vi "GUI_Cameras.vi"() -> ()   [LabVIEW 2020]
uses:
  Shared/GUI_Template/GUI_master/tcp_new_data_event.ctl
  Shared/GUI_Template/GUI_master/tcp new data cluster.ctl
  color tables/image color table presets.ctl
  Controls/Crosshair type def.ctl
  Controls/IMAQ control.ctl
  <vilib>/vision/Image Controls.llb/IMAQ Image.ctl
  Controls/Image Processing Controls.ctl
  Controls/GUI_running average centroid overlay.ctl
  Controls/Image Analysis Controls.ctl
  <vilib>/Utility/miscctls.llb/LVRectTypeDef.ctl
  <userlib>/_OpenG.lib/comparison/comparison.llb/Boolean Changed__ogtk.vi
  <vilib>/vision/NI_Vision_Development_Module.lvlib
panel:
  in  "stop":bool
  in  "Maximize!!":bool
  out "image::1":T1(plugin-control) caption="HPD_CCD"
  out "tcp data event":T2
  in  "Tab Control":T3(tab)
  out "Timestamp":timestamp format="%<%I:%M:%S%3u %p>T"
  in  "Max count":T4(ring)
  in  "Size & Tolerance":T5={"X Size"=5, "Y Size"=5, "% Tolerance"=100} {"Y Size" min=1 max=8; "X Size" min=1 max=8}
  in  "Clear ROI":bool caption="draw Xhair"
  in  "Set ROI":bool caption="draw Xhair"
  in  "LowPass":bool
  out "Max Counts":dbl(slide) scale=0.0..255.0
  in  "Color table":T6=enum."Rainbow"
  out "Rate (Hz)":sgl
  in  "analysis::1":bool caption="Analysis"
  in  "Scale":bool
  in  "Autoscale":bool
  in  "trigger::1":bool caption="Trigger"
  in  "save::1":bool caption="Save"
  in  "Scale":bool caption="Beep if Sat"
  in  "PerspectiveCorrectGUI::1":bool caption="Perspective"
  in  "roi.offsetY::1":u32 caption="ROI:OffsetY" max=1000
  in  "roi.offsetX::1":u32 caption="ROI:OffsetX" max=1000
  in  "roi.height::1":u32 caption="ROI:Height" min=1 max=3000
  in  "roi.width::1":u32 caption="ROI.Width" min=1 max=3000
  in  "SpatialCalibration::1":dbl caption="um/pix" min=0.0 max=9999999.0
  in  "Sat Level":sgl=255.0
  in  "triggerdelay::1":dbl caption="Triggerdelay" min=0.0 max=0.09
  in  "exposure::1":dbl=0.52 caption="Exposure" min=3.8e-05 max=1.0
  in  "gain::1":dbl caption="Gain" min=0.0 max=240.0
  in  "scale factor":dbl=2.0 caption="Scale factor"
  out "UDP error message":string caption="Device Errors"
  out "Perspective error":bool
  out "LastUpdate(s)":dbl format="%#_3g"
  in  "Type of Symmetry":T7(ring)
  in  "Rotate 2":bool caption="Flip"
  in  "Angle":dbl
  in  "Rotate":bool
  in  "BG Bit depth":string="12"
  in  "Subtract background":bool
  in  "BackgroundPath::1":path caption="BackgroundPath"
  in  "PerspectivePath::1":path caption="Perspective Calibration File Path"
  in  "AnalysisROITop::1":u32 caption="Top" max=2500
  in  "AnalysisROILeft::1":u32 caption="Left" max=2500
  in  "AnalysisROIBottom::1":u32 caption="Bottom" max=3000
  in  "AnalysisROIRight::1":u32 caption="Right" max=2500
  in  "Set Analysis ROI":bool caption="draw Xhair"
  in  "AnalysisROI::1":bool caption="AnalysisROI"
  in  "Draw From Centroid 2":bool=TRUE caption="draw Xhair"
  in  "Draw From\n Centroid 1":bool=TRUE caption="draw Xhair"
  in  "Crosshair.Label2::1":string="HPD_CCD" caption="CrosshairLabel2"
  in  "Crosshair.Label1::1":string="HPD_CCD" caption="CrosshairLabel1"
  in  "Target2.X::1":dbl caption="Target2X" min=0.0 max=2000.0
  in  "Target2.Y::1":dbl caption="Target2Y" min=0.0 max=2000.0
  in  "draw Xhair 2":bool caption="draw Xhair"
  in  "Target2Size.X::1":dbl=20.0 caption="Size2 x" min=0.0 max=2000.0
  in  "Target2Size.Y::1":dbl=20.0 caption="Size2 y" min=0.0 max=2000.0
  in  "Crosshair 2\nColor":u32(colorbox)=1250067
  in  "Crosshair 2Thickness":i32=1 caption="Crosshair 2\nThickness" min=0 max=2000
  in  "Overlay\nCentroid":T8={"draw Xhair 2"=FALSE, "Size x"=20.0, "Size y"=20.0, "# images to average"=20, "Centroid \nOverlay Color"=13435100} {"# images to average" min=0 max=2000; "Size y" min=0.0 max=2000.0; "Size x" min=0.0 max=2000.0}
  in  "Target.X::1":dbl caption="TargetX" min=0.0 max=2000.0
  in  "Target.Y::1":dbl caption="TargetY" min=0.0 max=2000.0
  in  "draw Xhair":bool=TRUE
  in  "TargetSize.X::1":dbl=20.0 caption="Size x" min=2.0 max=3000.0
  in  "TargetSize.Y::1":dbl=20.0 caption="Size y" min=2.0 max=3000.0
  in  "Crosshair\nColor":u32(colorbox)=1250067
  in  "Crosshair Thickness":i32=1 caption="Crosshair\nThickness" min=0 max=2000
  in  "GUI Crosshair":T9={"Draw"=FALSE, "Target"={"x"=0.0, "y"=0.0}, "Size"={"x"=20.0, "y"=20.0}, "Angle"=0.0, "Color"=1250067, "Thickness"=1, "CrosshairLabel"=""} {"Thickness" max=0; "Angle" format="%#_13g"; "Size"."y" min=0.0 max=0.0; "Size"."x" min=0.0 max=0.0}
  out "2ndmomW0y45::1":dbl caption="2ndmomW0y45" min=0.0 max=999999.0
  out "2ndmomW0x45::1":dbl caption="2ndmomW0x45" min=0.0 max=999999.0
  out "2ndmomW0y::1":dbl caption="2ndmomW0y" min=0.0 max=999999.0
  in  "Tab Control 2":enum32{"Mean", "Histogram", "Lineout"}(tab)
  out "Chart":dbl[][](graph)
  out "histogram":T10(graph)
  out "Mean Value":sgl format="%.2f"
  out "lineout":cluster{"x0":sgl, "dx":sgl, "Pixels Line":sgl[]}(graph)
  in  "GUI_Analysis":bool
  out "FWHMx (um)":dbl
  out "FWHMy (um)":dbl
  out "2ndmomW0x::1":dbl caption="2ndmomW0x" min=0.0 max=999999.0
  in  "FWHMx::1":dbl caption="FWHMx" min=0.0 max=999999.0
  in  "FWHMy::1":dbl caption="FWHMy" min=0.0 max=999999.0
  in  "centroidx::1":dbl caption="Centroidx" min=0.0 max=0.0
  in  "centroidy::1":dbl caption="Centroidy" min=0.0 max=0.0
  out "meancounts::1":dbl caption="MeanCounts" min=0.0 max=999999999.0
  in  "maxcounts::1":dbl caption="MaxCounts" min=0.0 max=999999999.0
  in  "acq_timestamp::1":dbl caption="acq_timestamp" min=0.0 max=0.0
  in  "localsavingpath::1":path caption="LocalSavingPath"
  in  "GUIdevice 1":string="HPD_CCD"
  in  "Hide controls":bool
  out "Current State":string
  out "ms since last display":u32
  out "process time":u32
  out "Custom Data Out":string
  out "Image Different?":bool
  in  "MeanCountsRaw::1":dbl caption="MeanCountsRaw" min=0.0 max=0.0
  out "Image (IMAQ)":T1(plugin-control)
  # "Set Crosshair\nto Centroid"
  # "Mean"
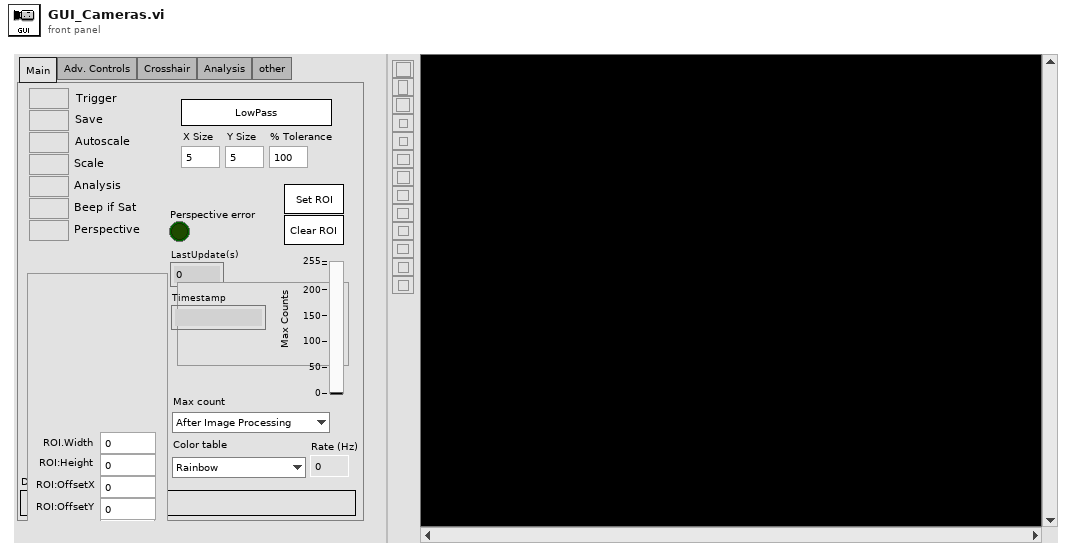
[diagram p1: front panel]
types:
  T1 = typedef "IMAQ Image.ctl" = refnum<image>
  T2 = typedef "tcp_new_data_event.ctl" = refnum<user-event>
  T3 = enum32{"Main", "Adv. Controls", "Crosshair", "Analysis", "other"}
  T4 = enum16{"After Image Processing", "Before Image Processing"}
  T5 = cluster{"X Size":i32, "Y Size":i32, "% Tolerance":i32}
  T6 = typedef "image color table presets.ctl" = enum16{"Greyscale", "Binary", "Gradient", "Rainbow", "Temperature", "enhance low", "blue yellow red", "BYR enhance low", "white blue yellow", "BWR enhance low", "make a new one"}
  T7 = enum16{"Horizontal", "Vertical", "Central", "1st Diagonal", "2nd Diagonal"}
  T8 = cluster{"draw Xhair 2":bool, "Size x":dbl, "Size y":dbl, "# images to average":i32, "Centroid \nOverlay Color":u32}
  T9 = typedef "Crosshair type def.ctl" = cluster{"Draw":bool, "Target":cluster{"x":dbl, "y":dbl}, "Size":cluster{"x":dbl, "y":dbl}, "Angle":dbl, "Color":u32, "Thickness":u8, "CrosshairLabel":string}
  T10 = cluster{"Starting Value":sgl, "Incremental Value":sgl, "Histogram":u32[]}
  T11 = enum32{"Invalid", "Standard", "Closed", "Hidden", "Minimized", "Maximized"}
  T12 = enum32{"invalid app kind", "Development System", "Run Time System", "Student Edition", "Embedded LabVIEW", "Evaluation", "Custom"}
  T13 = typedef "tcp new data cluster.ctl" = cluster{"EventEnum":enum16{"new data", "connection status update"}, "Device name":string}
  T14 = typedef "GUI_running average centroid overlay.ctl" = cluster{"CentroidX array":dbl[], "CentroidY array":dbl[], "CentroidX":dbl, "CentroidY":dbl, "# images to average":i32, "Crosshair":T9}
  T15 = cluster{"2ndmomW0y45::1":dbl, "2ndmomW0x45::1":dbl, "2ndmomW0y::1":dbl, "2ndmomW0x::1":dbl}
  T16 = cluster{"SpatialCalibration":dbl, "FWHMx":dbl, "FWHMy":dbl, "Analysis":bool}
  T17 = cluster{"LowPass":bool, "Size & Tolerance":cluster{"X Size":i32, "Y Size":i32, "% Tolerance":i32}}
  T18 = cluster{"Global Rectangle":i32[], "Contours":cluster{"Contour Type":u32, "ROI Type":u32, "Points":i32[]}[]}
  T19 = typedef "IMAQ Rectangle" = cluster{"Left":i32, "Top":i32, "Right":i32, "Bottom":i32, "Rotation":dbl}
  T20 = typedef "IMAQ control.ctl" = cluster{"Image SM":T1, "valid image":bool, "X resolution":i32, "Y resolution":i32, "Image Area":cluster{"Width":u32, "Height":u32}, "zoom to fit":bool, "Image Center":cluster{"X":u32, "Y":u32}, "Max count":dbl}
  T21 = typedef "Image Processing Controls.ctl" = cluster{"Crosshair IN":T9, "Autoscale":bool, "Scale":cluster{"scale factor":dbl, "Scale":bool}, "Lowpass IN":cluster{"LowPass":bool, "Size & Tolerance":cluster{"X Size":i32, "Y Size":i32, "% Tolerance":i32}}, "Image":T1, "GUI_centroid overlay":T14, "GUI Crosshair":T9, "Crosshair2 IN":T9, "calibration image":T1, "Perspective correection":bool, "Background image":T1, "Subtract background":bool, "Rotate Image":cluster{"Rotate":bool, "Rotation Angle":dbl}, "Flip Image":cluster{"Ring":u16, "Flip":bool}}
  T22 = typedef "Image Analysis Controls.ctl" = cluster{"Analysis":cluster{"IN":cluster{"SpatialCalibration":dbl, "FWHMx":dbl, "FWHMy":dbl, "Analysis":bool}, "OUT":cluster{"FWHMx (um)":dbl, "FWHMy (um)":dbl}}, "Histogram OUT":cluster{"histogram":cluster{"Starting Value":sgl, "Incremental Value":sgl, "Histogram":u32[]}, "Mean Value Graph":sgl, "Mean Value":sgl}, "Lineout":cluster{"IN":cluster{"ROI":cluster{"Global Rectangle":i32[], "Contours":cluster{"Contour Type":u32, "ROI Type":u32, "Points":i32[]}[]}}, "OUT":cluster{"lineout":cluster{"x0":sgl, "dx":sgl, "Pixels Line":sgl[]}, "Centroid":cluster{"X Centroid":sgl, "Y Centroid":sgl}, "Max Counts":cluster{"Max":sgl, "Color":u32}}}, "Image":T1, "variables":cluster{"2ndmomW0y45::1":dbl, "2ndmomW0x45::1":dbl, "2ndmomW0y::1":dbl, "2ndmomW0x::1":dbl}}
  T23 = typedef "LVRectTypeDef.ctl" = cluster{"Left":i16, "Top":i16, "Right":i16, "Bottom":i16}
  T24 = cluster{"Core":cluster{"Current VI Reference":refnum<vi>, "Close Panel on Exit?":bool}, "tcp connections":refnum<k5>[], "subscribe messages":string[], "Image Data":T20, "Image Process":T21, "Image Analysis":T22, "FP":cluster{"size":T23, "Resize Image":bool}, "Max count":dbl, "Max count before Image Processing":dbl, "Supergui":cluster{"image::1":T1, "STOP queue":refnum<queue>, "SuperGUI ref":refnum<vi>}, "Graph":dbl[][], "New Image":T1, "All Devices":string[], "PerspectivePath":path, "Old Timestamp":dbl}
  T25 = typedef "Image Type" = u32
  T26 = cluster{"image::1":T1, "STOP queue":refnum<queue>, "SuperGUI ref":refnum<vi>}
  T27 = cluster{"Current VI Reference":refnum<vi>, "Close Panel on Exit?":bool}
  T28 = cluster{"histogram":u32[], "Minimal Value":sgl, "Maximal Value":sgl, "Starting Value":sgl, "Interval Width":sgl, "Mean Value":sgl, "Standard  Variation":sgl, "Area (pixels)":i32}
  T29 = cluster{"TargetSize.X::1":dbl, "TargetSize.Y::1":dbl}
  T30 = cluster{"Target2Size.X::1":dbl, "Target2Size.Y::1":dbl}
  T31 = cluster{"Type of Symmetry":enum16{"Horizontal", "Vertical", "Central", "1st Diagonal", "2nd Diagonal"}, "Rotate 2":bool}
  T32 = cluster{"lineout":cluster{"x0":sgl, "dx":sgl, "Pixels Line":sgl[]}, "Centroid":cluster{"X Centroid":sgl, "Y Centroid":sgl}, "Max Counts":cluster{"Max":sgl, "Color":u32}}
  T33 = cluster{"histogram":cluster{"Starting Value":sgl, "Incremental Value":sgl, "Histogram":u32[]}, "Mean Value Graph":sgl, "Mean Value":sgl}
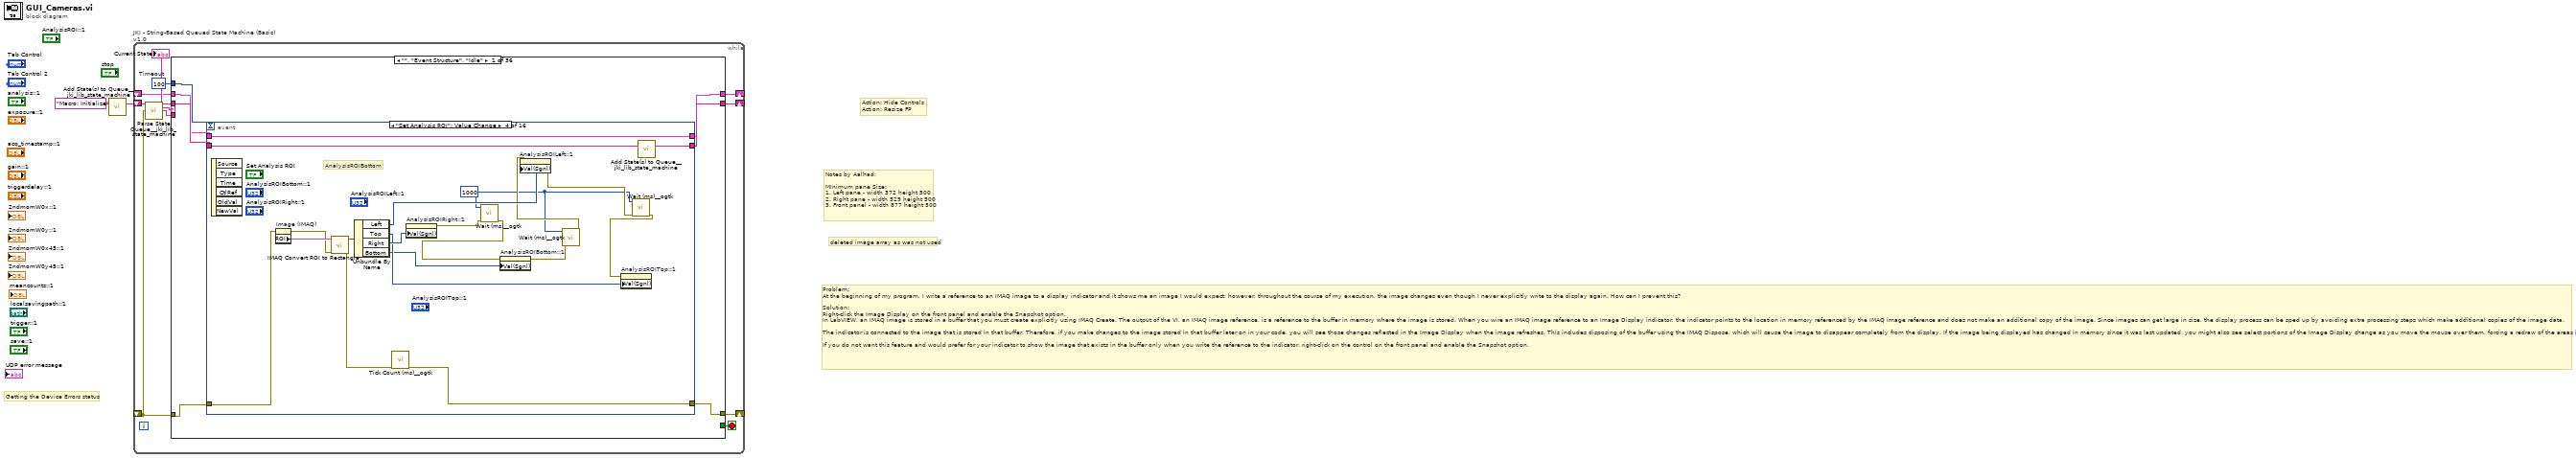
[diagram p0: block diagram]
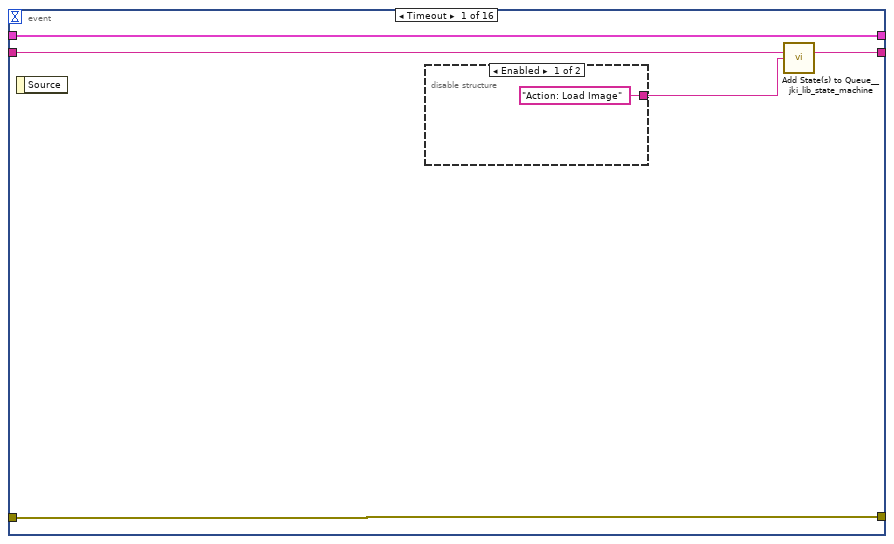
[diagram p2: hidden frame]
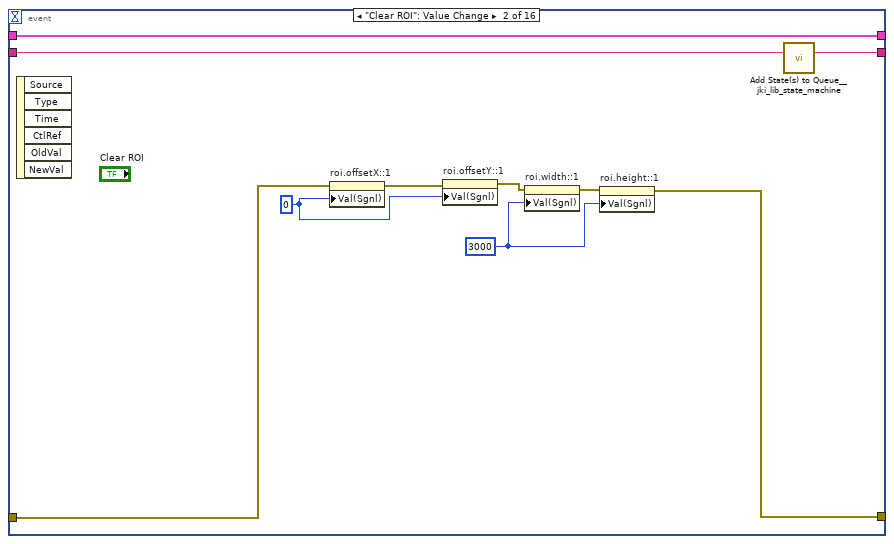
[diagram p4: hidden frame]
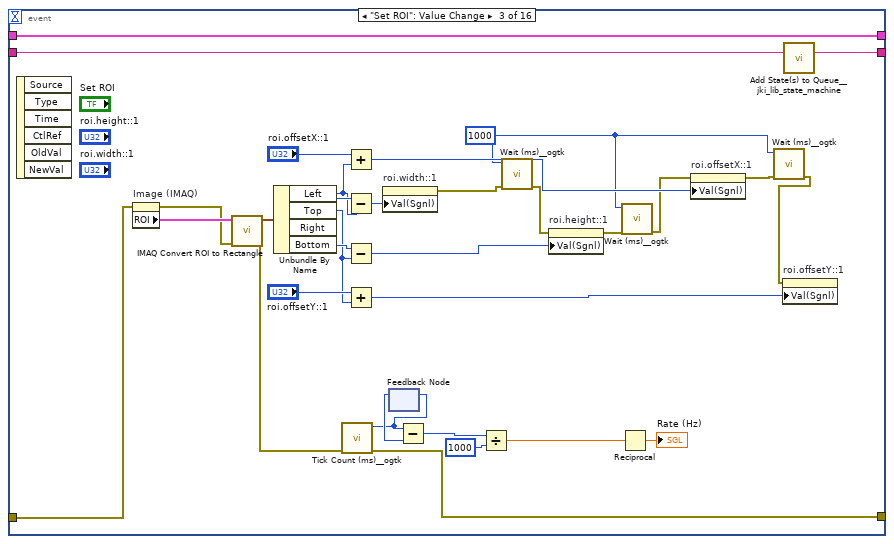
[diagram p5: hidden frame]
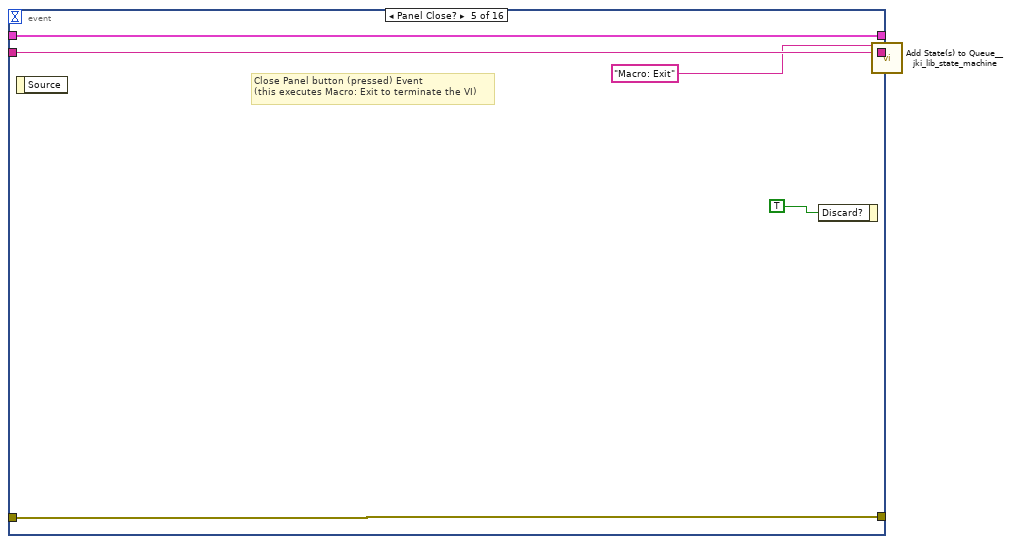
[diagram p6: hidden frame]
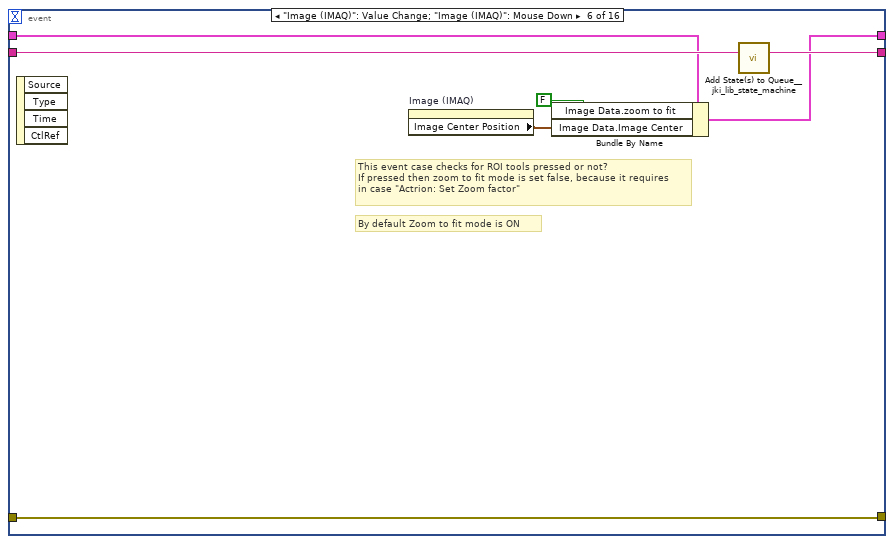
[diagram p7: hidden frame]
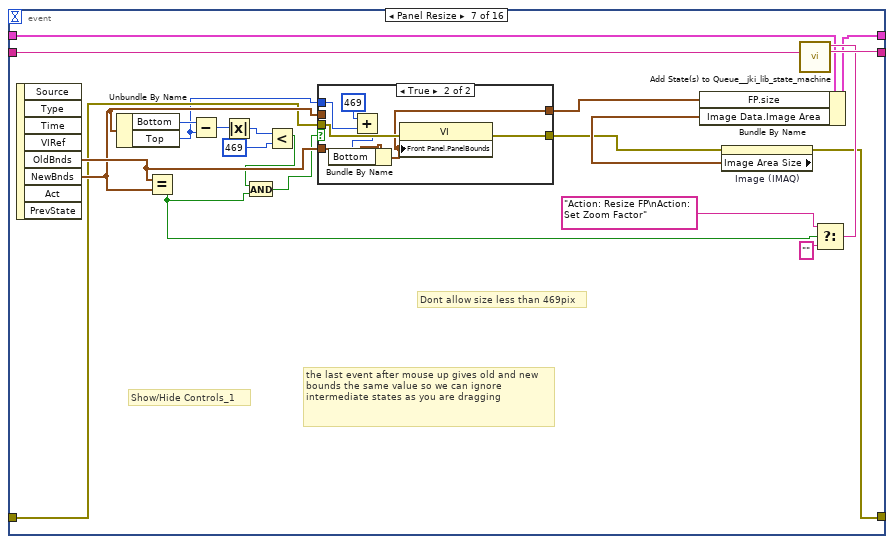
[diagram p8: hidden frame]
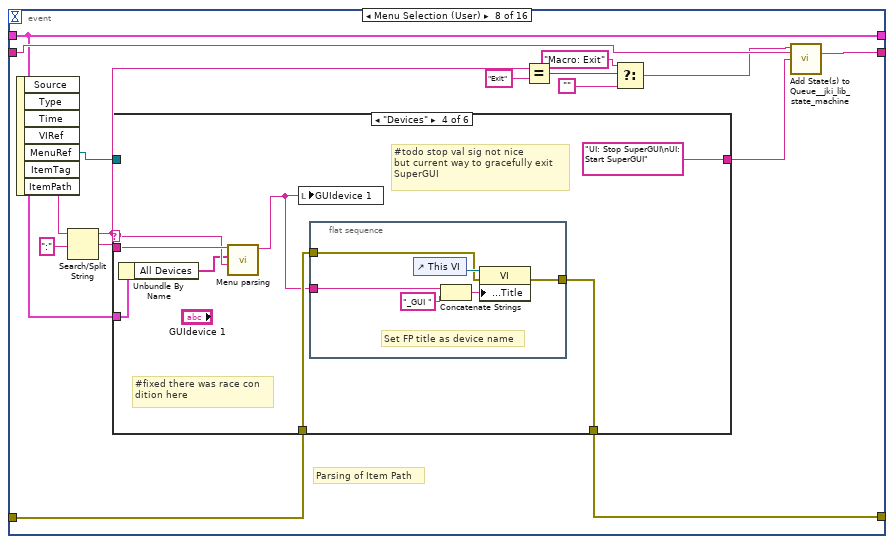
[diagram p10: hidden frame]
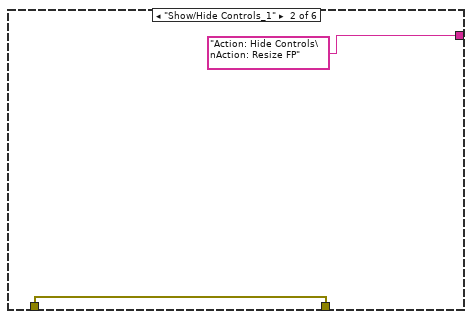
[diagram p12: hidden frame]
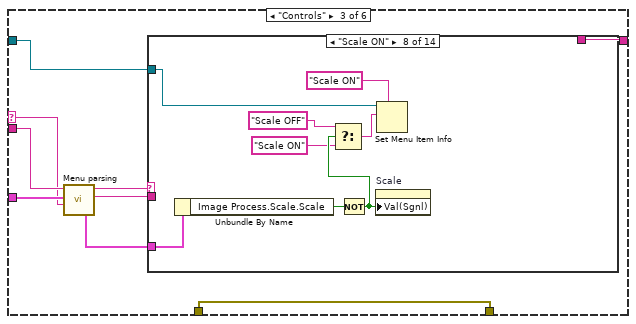
[diagram p13: hidden frame]
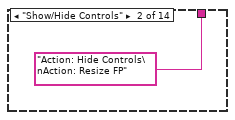
[diagram p15: hidden frame]
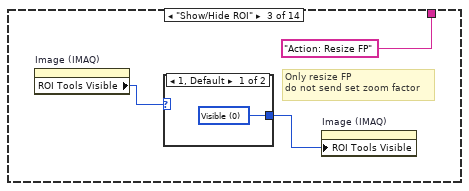
[diagram p16: hidden frame]
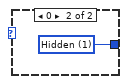
[diagram p17: hidden frame]
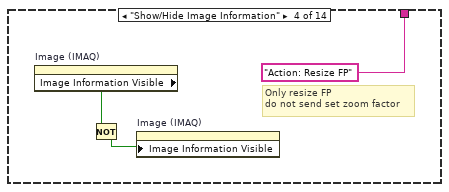
[diagram p18: hidden frame]
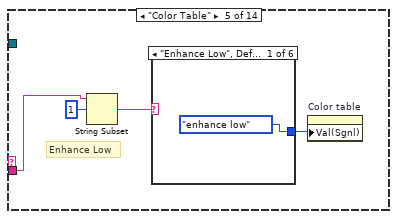
[diagram p19: hidden frame]
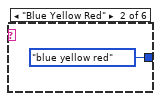
[diagram p20: hidden frame]
diagram:
  # "Getting the Device Errors status"
  # "Notes by Aalhad:\n\nMInimum pane Size:\n1. Left pane - width 372 height 500\n2. Right pane - width 529 height 500\n3. Front panel - width 877 height 500"
  # "deleted image array as was not used"
  # "Problem: \nAt the beginning of my program, I write a reference to an IMAQ image to a display indicator and it shows me an image I would expect; however, throughout the course of my execution, the image changes even though I never explicitly write to the display again. How can I prevent this?\n\nSolution: \nRight-click the Image Display on the front panel and enable the Snapshot option.\nIn LabVIEW, an IMAQ image is stored in a buffer that you must create explicitly using IMAQ Create. The output of the VI, an IMAQ image reference, is a reference to the buffer in memory where the image is stored. When you wire an IMAQ image reference to an Image Display indicator, the indicator points to the location in memory referenced by the IMAQ image reference and does not make an additional copy of the image. Since images can get large in size, the display process can be sped up by avoiding extra processing steps which make additional copies of the image data.\n\nThe indicator is connected to the image that is stored in that buffer. Therefore, if you make changes to the image stored in that buffer later on in your code, you will see those changes reflected in the Image Display when the image refreshes. This includes disposing of the buffer using the IMAQ Dispose, which will cause the image to disappear completely from the display. If the image being displayed has changed in memory since it was last updated, you might also see select portions of the Image Display change as you move the mouse over them, forcing a redraw of the areas it passes through.\n\nIf you do not want this feature and would prefer for your indicator to show the image that exists in the buffer only when you write the reference to the indicator, right-click on the control on the front panel and enable the Snapshot option."
  # "Action: Hide Controls\nAction: Resize FP"
  n1 = call <vilib>:"Add State(s) to Queue__jki_lib_state_machine.vi"("State(s) in (\"\")"="Macro: Initialize") -> ("States Out"=w2:string)  [unwired: 14 in]
  n2 = while "JKI - String-Based Queued State Machine (Basic) v1.0" {
    shift-right: [w6] -> _
    shift-left: _ -> [w5]
    shift-right: [w9] -> _
    shift-left: _ -> [w3]
    shift-right: [w8] -> _
    shift-left: w2 -> [w10]
    stop <- w7 stop-if-true
    w4 = 100  # Timeout
    n3 = call <vilib>:"Parse State Queue__jki_lib_state_machine.vi"("State Queue"=w10, "Error In (no error)"=w3) -> ("Remaining States"=w12:string, "Current State"=w13:string, "Arguments"=w11:string)  [unwired: 11 in]
    "Current State" <- w13
    n4 = case shown="\"\", \"Event Structure\", \"Idle\"" w13 {
      selector: w13 -> [_ _ w352 _ _ _ _ _ _ _ _ _ _ _ _ _ _ _ _ _ _ _ _ _ _ _ _ _ _ _ _ _ _ _ _ _]
      tunnel: w12 -> [w20 w351 w356 w374 w382 w397 w401 w428 w437 w444 w461 w473 w478 w514 w539 w570 w592 w602 w637 w642 w647 w659 w663 w671 w703 w740 w764 w805 w831 w901 w923 w952 w989 w1005 w1023 w1048]
      tunnel: w11 -> [_ _ _ _ _ _ _ _ _ _ _ _ _ _ _ _ w587 w597 _ _ _ _ _ _ _ _ _ _ _ _ _ _ _ _ _ _]
      tunnel: w5 -> [w18 w348 w354 w366 w380 w395 w398 _ w434 w441 w455 w468 w479 w515 w538 w553 w590 w598 w634 w639 w644 w657 w660 w664 w697 w725 w771 w804 w835 w862 w921 w944 w972 w1006 w1020 w1037]
      tunnel: [w17 w349 w358 w371 w375 w394 w399 w425 w431 w442 w459 w462 w476 w511 w534 w557 w588 w599 w635 w640 w645 w651 w661 w665 w699 w727 w765 w807 w836 w900 w922 w930 w966 w1002 w1017 w1029] -> w9
      tunnel: w3 -> [w16 w349 w357 w371 w376 w394 w399 w425 w430 w442 w459 w469 w477 w512 w533 w554 w589 w600 w635 w640 w645 w651 w661 w669 w701 w734 w766 w824 w833 w900 w922 w948 w965 w1003 w1018 w1027]
      tunnel: [w19 w350 w355 w373 w381 w396 w400 w427 w436 w443 w460 w473 w478 w514 w539 w570 w591 w601 w636 w641 w646 w658 w662 w670 w702 w739 w763 w806 w831 w901 w923 w952 w989 w1005 w1023 w1047] -> w8
      tunnel: [_ _ _ _ _ TRUE _ _ _ _ _ _ _ _ _ _ _ _ _ _ _ _ _ _ _ _ _ _ _ _ _ _ _ _ _ _] -> w7
      tunnel: [w15 w348 w354 w372 w380 w395 w398 w426 w434 w441 w454 w467 w479 w515 w538 w556 w590 w598 w634 w639 w644 w657 w660 w668 w700 w726 w770 w803 w834 w899 w920 w949 w972 w1006 w1020 w1037] -> w6
      tunnel: w4 -> [w14 _ _ _ _ _ _ _ _ _ _ _ _ _ _ _ _ _ _ _ _ _ _ _ _ _ _ _ _ _ _ _ _ _ _ _]
      frame "", "Event Structure", "Idle" {
        n5 = event shown="[3] \"Set Analysis ROI\": Value Change" {
          selector: _ -> [_ _ _ _ _ _ _ _ _ _ _ _ _ _ _ _]
          dyn-events: _ -> [_ _ _ _ _ _ _ _ _ _ _ _ _ _ _ _]
          timeout: w14 -> [_ _ _ _ _ _ _ _ _ _ _ _ _ _ _ _]
          tunnel: w20 -> [w25 w36 w68 w88 w94 w100 w122 w140 w280 w298 w304 w309 w315 w331 w339 w347]
          tunnel: [w24 w35 w67 w87 w93 w101 w123 w138 w279 w297 w303 w309 w315 w331 w339 w347] -> w19
          tunnel: w18 -> [w21 w34 w66 w86 w91 w99 w118 w133 w286 w300 w306 w310 w316 w326 w337 w345]
          tunnel: [w23 w27 w44 w77 w92 w98 w106 w135 w281 w299 w305 w308 w311 w330 w338 w346] -> w17
          tunnel: w16 -> [w23 w28 w45 w78 w92 w98 w107 w136 w282 w299 w305 w308 w312 w330 w338 w346]
          tunnel: [w21 w34 w66 w86 w91 w97 w117 w133 w286 w300 w306 w310 w316 w325 w337 w345] -> w15
          event Timeout {
            n6 = event-data() -> ()  [unwired: 1 in, 1 out]
            n7 = disable-structure shown="Enabled" {
              disable-tunnel: ["Action: Load Image" ("State(s) in Front (\"\")") _] -> w22
              frame Enabled {
              }
              frame Disabled {
              }
            }
            n8 = call <vilib>:"Add State(s) to Queue__jki_lib_state_machine.vi"("State(s) in (\"\")"=w25, "State(s) at Back (\"\")"=w22) -> ("States Out"=w24:string)  [unwired: 13 in]
          }
          event "Clear ROI": Value Change {
            w31 = 3000
            w33 = 0
            n9 = event-data() -> ()  [unwired: 1 in, 6 out]
            n10 = property on="roi.offsetX::1" class="DigNum (strict)"(error in=w28, "Val(Sgnl)"=w33) -> (error out=w32:errorcluster)  [unwired: 1 in, 1 out]
            n11 = property on="roi.offsetY::1" class="DigNum (strict)"(error in=w32, "Val(Sgnl)"=w33) -> (error out=w30:errorcluster)  [unwired: 1 in, 1 out]
            n12 = property on="roi.width::1" class="DigNum (strict)"(error in=w30, "Val(Sgnl)"=w31) -> (error out=w29:errorcluster)  [unwired: 1 in, 1 out]
            n13 = property on="roi.height::1" class="DigNum (strict)"(error in=w29, "Val(Sgnl)"=w31) -> (error out=w27:errorcluster)  [unwired: 1 in, 1 out]
            n14 = call <vilib>:"Add State(s) to Queue__jki_lib_state_machine.vi"("State(s) in (\"\")"=w36) -> ("States Out"=w35:string)  [unwired: 14 in]
          }
          event "Set ROI": Value Change {
            w38 = u32 1000 ("milliseconds to wait")
            n15 = event-data() -> ()  [unwired: 1 in, 6 out]
            n16 = property on="Image (IMAQ)" class="ImageControl"(error in=w45) -> (error out=w47:errorcluster, "ROI"=w64:T18)  [unwired: 1 in, 1 out]
            n17 = call "IMAQ Convert ROI to Rectangle"("error in (no error)"=w47, "ROI Descriptor"=w64) -> ("error out"=w46:errorcluster, "Rectangle"=w65:T19)  [unwired: 7 in]
            n18 = Unbundle By Name(w65) -> ("Left"=w58:i32, "Top"=w55:i32, "Right"=w59:i32, "Bottom"=w56:i32)
            n19 = call <userlib>:"Tick Count (ms)__ogtk.vi"("error in (no error)"=w46) -> ("error out"=w44:errorcluster, "millisecond timer value"=w52:u32)  [unwired: 9 in]
            n20 = Add(x="roi.offsetX::1", y=w58) -> (x+y=w62:u32)
            n21 = Subtract(x=w59, y=w58) -> (x-y=w57:i32)
            n22 = Subtract(x=w56, y=w55) -> (x-y=w54:i32)
            n23 = Add(x="roi.offsetY::1", y=w55) -> (x+y=w60:u32)
            n24 = property on="roi.width::1" class="DigNum (strict)"("Val(Sgnl)"=w57) -> (error out=w43:errorcluster)  [unwired: 2 in, 1 out]
            n25 = feedback #1() -> (w53:u32)  [unwired: 1 in]
            n26 = feedback-in #1(w52) -> ()
            n27 = Subtract(x=w52, y=w53) -> (x-y=w51:u32)
            n28 = Divide(x=w51, y=u32 1000) -> (x/y=w49:dbl)
            n29 = call <userlib>:"Wait (ms)__ogtk.vi"("error in (no error)"=w43, "milliseconds to wait"=w38) -> ("error out"=w42:errorcluster)  [unwired: 8 in, 1 out]
            n30 = property on="roi.height::1" class="DigNum (strict)"(error in=w42, "Val(Sgnl)"=w54) -> (error out=w41:errorcluster)  [unwired: 1 in, 1 out]
            n31 = Reciprocal(x=w49) -> (1/x=→"Rate (Hz)":dbl)
            n32 = call <userlib>:"Wait (ms)__ogtk.vi"("error in (no error)"=w41, "milliseconds to wait"=w38) -> ("error out"=w40:errorcluster)  [unwired: 8 in, 1 out]
            n33 = property on="roi.offsetX::1" class="DigNum (strict)"(error in=w40, "Val(Sgnl)"=w62) -> (error out=w39:errorcluster)  [unwired: 1 in, 1 out]
            n34 = call <userlib>:"Wait (ms)__ogtk.vi"("error in (no error)"=w39, "milliseconds to wait"=w38) -> ("error out"=w37:errorcluster)  [unwired: 8 in, 1 out]
            n35 = property on="roi.offsetY::1" class="DigNum (strict)"(error in=w37, "Val(Sgnl)"=w60) -> ()  [unwired: 1 in, 2 out]
            n36 = call <vilib>:"Add State(s) to Queue__jki_lib_state_machine.vi"("State(s) in (\"\")"=w68) -> ("States Out"=w67:string)  [unwired: 14 in]
          }
          event "Set Analysis ROI": Value Change {
            w71 = u32 1000 ("milliseconds to wait")
            # "AnalysisROIBottom"
            n37 = event-data() -> ()  [unwired: 1 in, 6 out]
            n38 = property on="Image (IMAQ)" class="ImageControl"(error in=w78) -> (error out=w80:errorcluster, "ROI"=w84:T18)  [unwired: 1 in, 1 out]
            n39 = call "IMAQ Convert ROI to Rectangle"("error in (no error)"=w80, "ROI Descriptor"=w84) -> ("error out"=w79:errorcluster, "Rectangle"=w85:T19)  [unwired: 7 in]
            n40 = Unbundle By Name(w85) -> ("Left"=w82:i32, "Top"=w81:i32, "Right"=w83:i32, "Bottom"=w69:i32)
            n41 = call <userlib>:"Tick Count (ms)__ogtk.vi"("error in (no error)"=w79) -> ("error out"=w77:errorcluster)  [unwired: 9 in, 1 out]
            n42 = property on="AnalysisROIRight::1" class="DigNum (strict)"("Val(Sgnl)"=w83) -> (error out=w76:errorcluster)  [unwired: 2 in, 1 out]
            n43 = call <userlib>:"Wait (ms)__ogtk.vi"("error in (no error)"=w76, "milliseconds to wait"=w71) -> ("error out"=w75:errorcluster)  [unwired: 8 in, 1 out]
            n44 = property on="AnalysisROIBottom::1" class="DigNum (strict)"(error in=w75, "Val(Sgnl)"=w69) -> (error out=w74:errorcluster)  [unwired: 1 in, 1 out]
            n45 = call <userlib>:"Wait (ms)__ogtk.vi"("error in (no error)"=w74, "milliseconds to wait"=w71) -> ("error out"=w73:errorcluster)  [unwired: 8 in, 1 out]
            n46 = property on="AnalysisROILeft::1" class="DigNum (strict)"(error in=w73, "Val(Sgnl)"=w82) -> (error out=w72:errorcluster)  [unwired: 1 in, 1 out]
            n47 = call <userlib>:"Wait (ms)__ogtk.vi"("error in (no error)"=w72, "milliseconds to wait"=w71) -> ("error out"=w70:errorcluster)  [unwired: 8 in, 1 out]
            n48 = property on="AnalysisROITop::1" class="DigNum (strict)"(error in=w70, "Val(Sgnl)"=w81) -> ()  [unwired: 1 in, 2 out]
            n49 = call <vilib>:"Add State(s) to Queue__jki_lib_state_machine.vi"("State(s) in (\"\")"=w88) -> ("States Out"=w87:string)  [unwired: 14 in]
          }
          event Panel Close? {
            # "Close Panel button (pressed) Event\n(this executes Macro: Exit to terminate the VI)"
            n50 = event-data() -> ()  [unwired: 1 in, 1 out]
            n51 = event-data("Discard?"=TRUE) -> ()  [unwired: 1 in, 1 out]
            n52 = call <vilib>:"Add State(s) to Queue__jki_lib_state_machine.vi"("State(s) in Front (\"\")"="Macro: Exit", "State(s) in (\"\")"=w94) -> ("States Out"=w93:string)  [unwired: 13 in]
          }
          event "Image (IMAQ)": Value Change; "Image (IMAQ)": Mouse Down {
            # "By default Zoom to fit mode is ON"
            # "This event case checks for ROI tools pressed or not?\nIf pressed then zoom to fit mode is set false, because it requires\nin case \"Actrion: Set Zoom factor\""
            n53 = event-data() -> ()  [unwired: 1 in, 4 out]
            n54 = property on="Image (IMAQ)" class="ImageControl"() -> ("Image Center Position"=w96:cluster{"X":u32, "Y":u32})  [unwired: 2 in, 2 out]
            n55 = Bundle By Name(cluster=w99, "Image Data.zoom to fit"=FALSE, "Image Data.Image Center"=w96) -> (w97:T24)
            n56 = call <vilib>:"Add State(s) to Queue__jki_lib_state_machine.vi"("State(s) in (\"\")"=w100) -> ("States Out"=w101:string)  [unwired: 14 in]
          }
          event Panel Resize {
            # "Dont allow size less than 469pix"
            # "Show/Hide Controls_1"
            # "the last event after mouse up gives old and new bounds the same value so we can ignore intermediate states as you are dragging"
            n57 = event-data() -> ("OldBnds"=w111:T23, "NewBnds"=w109:T23)  [unwired: 1 in, 6 out]
            n58 = Unbundle By Name(w109) -> ("Bottom"=w115:i16, "Top"=w103:i16)
            n59 = Equal?(x=w111, y=w109) -> (x = y?=w102:bool)
            n60 = Subtract(x=w115, y=w103) -> (x-y=w114:i16)
            n61 = Absolute Value(x=w114) -> (abs(x)=w113:i16)
            n62 = Less?(x=w113, y=i16 469) -> (x < y?=w105:bool)
            n63 = And(x=w105, y=w102) -> (x .and. y?=w104:bool)
            n64 = case shown="True" w104 {
              tunnel: w111 -> [_ w130]
              tunnel: [w125 w126] -> w110
              tunnel: w109 -> [w125 _]
              tunnel: [w124 w132] -> w108
              tunnel: w107 -> [w124 w131]
              tunnel: w103 -> [_ w129]
              frame False {
              }
              frame True {
                n65 = Add(x=i16 469 ("y"), y=w129) -> (x+y=w127:i16)
                n66 = Bundle By Name(cluster=w130, "Bottom"=w127) -> (w126:T23)
                n67 = property class="VI"(error in=w131, "Front Panel.PanelBounds"=w126) -> (error out=w132:errorcluster)  [unwired: 1 in, 1 out]
              }
            }
            n68 = property on="Image (IMAQ)" class="ImageControl"(error in=w108) -> (error out=w106:errorcluster, "Image Area Size"=w116:cluster{"Width":u32, "Height":u32})  [unwired: 1 in, 1 out]
            n69 = Bundle By Name(cluster=w118, "FP.size"=w110, "Image Data.Image Area"=w116) -> (w117:T24)
            n70 = Select(t="Action: Resize FP\nAction: Set Zoom Factor" ("State(s) in Front (\"\")"), s=w102, f="" ("t")) -> (s? t:f=w119:string)
            n71 = call <vilib>:"Add State(s) to Queue__jki_lib_state_machine.vi"("State(s) in Front (\"\")"=w119, "State(s) in (\"\")"=w122) -> ("States Out"=w123:string)  [unwired: 13 in]
          }
          event Menu Selection (User) {
            # "Parsing of Item Path"
            n72 = event-data() -> ("MenuRef"=w146:refnum<k9>, "ItemPath"=w148:string)  [unwired: 1 in, 5 out]
            n73 = Search/Split String(string=w148, search string/char (-)=":") -> (substring before match=w137:string, match + rest of string=w145:string)  [unwired: 1 in, 1 out]
            n74 = case shown="\"Devices\"" w137 {
              selector: w137 -> [_ _ w152 w253 _ _]
              tunnel: w145 -> [_ _ w158 w258 _ _]
              tunnel: w146 -> [_ _ w159 _ _ _]
              tunnel: w133 -> [_ _ w155 w252 _ _]
              tunnel: w136 -> [w149 w151 w154 w257 w265 w268]
              tunnel: [w149 w151 w154 w256 w265 w267] -> w135
              tunnel: [_ "Action: Hide Controls\nAction: Resize FP" w153 "UI: Stop SuperGUI\nUI: Start SuperGUI" _ _] -> w134
              frame "", Default {
              }
              frame "Show/Hide Controls_1" {
              }
              frame "Controls" {
                n75 = call "Menu parsing.vi"("Menu Item"=w152, "ItemPath"=w158) -> ("Item Path 2"=w156:string, "ItemPath"=w157:string)  [unwired: 8 in]
                n76 = case shown="\"Scale ON\"" w157 {
                  tunnel: w159 -> [_ _ _ _ _ w182 w188 w201 w202 w211 w227 w235 w243 w250]
                  tunnel: w156 -> [_ _ _ _ w170 _ _ _ _ _ _ _ _ _]
                  tunnel: w155 -> [_ _ _ _ _ _ w187 w200 _ _ w225 w230 w240 _]
                  tunnel: [_ "Action: Hide Controls\nAction: Resize FP" "Action: Resize FP" "Action: Resize FP" _ _ _ _ _ _ _ _ _ _] -> w153
                  frame Default {
                  }
                  frame "Show/Hide Controls" {
                  }
                  frame "Show/Hide ROI" {
                    # "Only resize FP\ndo not send set zoom factor"
                    n77 = property on="Image (IMAQ)" class="ImageControl"() -> ("ROI Tools Visible"=w161:u32)  [unwired: 2 in, 2 out]
                    n78 = case shown="1, Default" w161 {
                      tunnel: [w164 w165] -> w163
                      frame 1, Default {
                        w164 = u32 0 items=["Visible", "Hidden", "Hidden, Use WindTools Palette"] ("ROI Tools Visible")
                      }
                      frame 0 {
                        w165 = u32 1 items=["Visible", "Hidden", "Hidden, Use WindTools Palette"] ("ROI Tools Visible")
                      }
                    }
                    n79 = property on="Image (IMAQ)" class="ImageControl"("ROI Tools Visible"=w163) -> ()  [unwired: 2 in, 2 out]
                  }
                  frame "Show/Hide Image Information" {
                    # "Only resize FP\ndo not send set zoom factor"
                    n80 = property on="Image (IMAQ)" class="ImageControl"() -> ("Image Information Visible"=w167:bool)  [unwired: 2 in, 2 out]
                    n81 = Not(x=w167) -> (.not. x?=w166:bool)
                    n82 = property on="Image (IMAQ)" class="ImageControl"("Image Information Visible"=w166) -> ()  [unwired: 2 in, 2 out]
                  }
                  frame "Color Table" {
                    # "Enhance Low"
                    n83 = String Subset(string=w170, offset (0)=1) -> (substring=w169:string)  [unwired: 1 in]
                    n84 = case shown="\"Enhance Low\", Default" w169 {
                      tunnel: [image_color_table_presets."enhance low" ("Value (Signaling)") image_color_table_presets."blue yellow red" ("Value (Signaling)") image_color_table_presets."BYR enhance low" ("Value (Signaling)") image_color_table_presets."white blue yellow" ("Value (Signaling)") image_color_table_presets."BWR enhance low" ("Value (Signaling)") image_color_table_presets."make a new one" ("Value (Signaling)")] -> w172
                      frame "Enhance Low", Default {
                      }
                      frame "Blue Yellow Red" {
                      }
                      frame "BYR enhance low" {
                      }
                      frame "White Blue Yellow" {
                      }
                      frame "BWR enhance low" {
                      }
                      frame "Make a new one" {
                      }
                    }
                    n85 = property on="Color table" class="Enum (strict)"("Val(Sgnl)"=w172) -> ()  [unwired: 2 in, 2 out]
                  }
                  frame "Maximize ON" {
                    n86 = local read "Maximize!!"() -> (w185:bool)
                    n87 = Not(x=w185) -> (.not. x?=w184:bool)
                    n88 = property on="Maximize!!" class="Bool (strict)"("Val(Sgnl)"=w184) -> ()  [unwired: 2 in, 2 out]
                    n89 = Select(t="Maximize OFF" ("item name"), s=w184, f="Maximize ON" ("item name")) -> (s? t:f=w180:string)
                    n90 = Set Menu Item Info(7:"Maximize ON" ("item tag"), 10:w180, 11:w182) -> ()  [unwired: 4 in, 2 out]
                  }
                  frame "Autoscale ON" {
                    n91 = Unbundle By Name(w187) -> ("Image Process.Autoscale"=w186:bool)
                    n92 = Not(x=w186) -> (.not. x?=w193:bool)
                    n93 = Select(t="Autoscale OFF" ("item name"), s=w193, f="Autoscale ON" ("item name")) -> (s? t:f=w189:string)
                    n94 = property on="Autoscale" class="Bool (strict)"("Val(Sgnl)"=w193) -> ()  [unwired: 2 in, 2 out]
                    n95 = Set Menu Item Info(7:"Autoscale ON" ("item tag"), 10:w189, 11:w188) -> ()  [unwired: 4 in, 2 out]
                  }
                  frame "Scale ON" {
                    n96 = Unbundle By Name(w200) -> ("Image Process.Scale.Scale"=w199:bool)
                    n97 = Not(x=w199) -> (.not. x?=w197:bool)
                    n98 = Select(t="Scale OFF" ("item name"), s=w197, f="Scale ON" ("item name")) -> (s? t:f=w194:string)
                    n99 = property on="Scale" class="Bool (strict)"("Val(Sgnl)"=w197) -> ()  [unwired: 2 in, 2 out]
                    n100 = Set Menu Item Info(7:"Scale ON" ("item tag"), 10:w194, 11:w201) -> ()  [unwired: 4 in, 2 out]
                  }
                  frame "Trigger ON" {
                    n101 = local read "trigger::1"() -> (w204:bool)
                    n102 = Not(x=w204) -> (.not. x?=w203:bool)
                    n103 = case shown="False" w203 {
                      tunnel: w202 -> [w206 w209]
                      frame True {
                        n104 = Set Menu Item Info(7:"Trigger ON" ("item tag"), 10:"Trigger OFF" ("item name"), 11:w206) -> ()  [unwired: 4 in, 2 out]
                      }
                      frame False {
                        n105 = Set Menu Item Info(7:"Trigger ON" ("item tag"), 10:"Trigger ON" ("item name"), 11:w209) -> ()  [unwired: 4 in, 2 out]
                      }
                    }
                    n106 = property on="trigger::1" class="Bool (strict)"("Val(Sgnl)"=w203) -> ()  [unwired: 2 in, 2 out]
                  }
                  frame "Save ON" {
                    n107 = local read "save::1"() -> (w213:bool)
                    n108 = Not(x=w213) -> (.not. x?=w212:bool)
                    n109 = case shown="True" w212 {
                      tunnel: w211 -> [w215 w218]
                      frame True {
                        n110 = Set Menu Item Info(7:"Save ON" ("item tag"), 10:"Save OFF" ("item name"), 11:w215) -> ()  [unwired: 4 in, 2 out]
                      }
                      frame False {
                        n111 = Set Menu Item Info(7:"Save ON" ("item tag"), 10:"Save ON" ("item name"), 11:w218) -> ()  [unwired: 4 in, 2 out]
                      }
                    }
                    n112 = property on="save::1" class="Bool (strict)"("Val(Sgnl)"=w212) -> ()  [unwired: 2 in, 2 out]
                  }
                  frame "Draw Crosshair ON" {
                    n113 = Unbundle By Name(w225) -> ("Image Process.Crosshair IN.Draw"=w224:bool)
                    n114 = Not(x=w224) -> (.not. x?=w221:bool)
                    n115 = Select(t="Draw Crosshair OFF" ("item name"), s=w221, f="Draw Crosshair ON" ("item name")) -> (s? t:f=w220:string)
                    n116 = Set Menu Item Info(7:"Draw Crosshair ON" ("item tag"), 10:w220, 11:w227) -> ()  [unwired: 4 in, 2 out]
                    n117 = property on="draw Xhair" class="Bool (strict)"("Val(Sgnl)"=w221) -> ()  [unwired: 2 in, 2 out]
                  }
                  frame "Low Pass ON" {
                    n118 = Unbundle By Name(w230) -> ("Image Process.Lowpass IN.LowPass"=w229:bool)
                    n119 = Not(x=w229) -> (.not. x?=w231:bool)
                    n120 = Select(t="Low Pass OFF" ("item name"), s=w231, f="Low Pass ON" ("item name")) -> (s? t:f=w228:string)
                    n121 = Set Menu Item Info(7:"Low Pass ON" ("item tag"), 10:w228, 11:w235) -> ()  [unwired: 4 in, 2 out]
                    n122 = property on="LowPass" class="Bool (strict)"("Val(Sgnl)"=w231) -> ()  [unwired: 2 in, 2 out]
                  }
                  frame "Analysis ON" {
                    n123 = Unbundle By Name(w240) -> ("Image Analysis.Analysis.IN.Analysis"=w239:bool)
                    n124 = Not(x=w239) -> (.not. x?=w241:bool)
                    n125 = Select(t="Analysis OFF" ("item name"), s=w241, f="Analysis ON" ("item name")) -> (s? t:f=w236:string)
                    n126 = Set Menu Item Info(7:"Analysis ON" ("item tag"), 10:w236, 11:w243) -> ()  [unwired: 4 in, 2 out]
                    n127 = property on="GUI_Analysis" class="Bool (strict)"("Val(Sgnl)"=w241) -> ()  [unwired: 2 in, 2 out]
                  }
                  frame "Beep If Saturation ON" {
                    n128 = local read "Scale"() -> (w244:bool)
                    n129 = Not(x=w244) -> (.not. x?=w248:bool)
                    n130 = Select(t="Beep If Saturation OFF" ("item name"), s=w248, f="Beep If Saturation ON" ("item name")) -> (s? t:f=w245:string)
                    n131 = Set Menu Item Info(7:"Beep If Saturation ON" ("item tag"), 10:w245, 11:w250) -> ()  [unwired: 4 in, 2 out]
                    n132 = property on="Scale" class="Bool (strict)"("Val(Sgnl)"=w248) -> ()  [unwired: 2 in, 2 out]
                  }
                }
              }
              frame "Devices" {
                # "#fixed there was race con\ndition here"
                # "#todo stop val sig not nice\nbut current way to gracefully exit\nSuperGUI"
                n133 = Unbundle By Name(w252) -> ("All Devices"=w251:string[])
                n134 = call "Menu parsing.vi"("Menu Item"=w253, "All devices"=w251, "ItemPath"=w258) -> ("ItemPath"=w254:string)  [unwired: 7 in, 1 out]
                n135 = local write "GUIdevice 1"(w254) -> ()
                n136 = flat-sequence {
                  tunnel: [w261] -> w256
                  tunnel: w257 -> [w260]
                  tunnel: w254 -> [w259]
                  frame #0 {
                    # "Set FP title as device name"
                    n137 = control-ref of="This VI"() -> (w264:refnum<vi>)
                    n138 = Concatenate Strings(w259, "_GUI ") -> (w263:string)
                    n139 = property class="VI"(reference=w264, error in=w260, "Front Panel.Title"=w263) -> (error out=w261:errorcluster)  [unwired: 1 out]
                  }
                }
              }
              frame "Exit" {
              }
              frame "Local Saving Path" {
                n140 = control-ref of="localsavingpath::1"() -> (w269:refnum<vi>)
                n141 = property class="Path"(reference=w269, error in=w268) -> (reference out=w271:refnum<vi>, error out=w266:errorcluster, "Value"=w270:path)
                n142 = call "changePath.vi"("Local Saving in (h)"=w270) -> ("change (h)"=w272:bool, "Local Saving out (h)"=w273:path)  [unwired: 9 in]
                n143 = case shown="True" w272 {
                  tunnel: w271 -> [_ w278]
                  tunnel: w273 -> [_ w277]
                  tunnel: [w274 w276] -> w267
                  tunnel: w266 -> [w274 w275]
                  frame False {
                  }
                  frame True {
                    n144 = property class="Path"(reference=w278, error in=w275, "Val(Sgnl)"=w277) -> (error out=w276:errorcluster)  [unwired: 1 out]
                  }
                }
              }
            }
            n145 = Equal?(x=w137, y="Exit") -> (x = y?=w143:bool)
            n146 = Select(t="Macro: Exit", s=w143, f="") -> (s? t:f=w139:string)
            n147 = call <vilib>:"Add State(s) to Queue__jki_lib_state_machine.vi"("State(s) in Front (\"\")"=w139, "State(s) in (\"\")"=w140, "State(s) at Back (\"\")"=w134) -> ("States Out"=w138:string)  [unwired: 12 in]
          }
          event "Maximize!!": Value Change {
            n148 = event-data() -> ()  [unwired: 1 in, 6 out]
            n149 = property class="VI"(error in=w282) -> (error out=w284:errorcluster, "Front Panel.PanelBounds"=w285:T23)  [unwired: 1 in, 1 out]
            n150 = case shown="True" "Maximize!!" {
              tunnel: w285 -> [w290 w294]
              tunnel: [w290 w294] -> _
              tunnel: [w287 w293] -> w281
              tunnel: w284 -> [w288 w291]
              frame False {
                n151 = property class="VI"(error in=w288, "Front Panel Window:State"=T11."Standard") -> (error out=w287:errorcluster)  [unwired: 1 in, 1 out]
              }
              frame True {
                n152 = property class="VI"(error in=w291, "Front Panel Window:State"=T11."Maximized") -> (error out=w293:errorcluster)  [unwired: 1 in, 1 out]
                n153 = Wait (ms)(milliseconds to wait=u32 200) -> ()  [unwired: 1 out]
              }
            }
            n154 = call <vilib>:"Add State(s) to Queue__jki_lib_state_machine.vi"("State(s) in (\"\")"=w280) -> ("States Out"=w279:string)  [unwired: 14 in]
          }
          event Value Change {
            n155 = event-data() -> ()  [unwired: 1 in, 6 out]
            n156 = call <vilib>:"Add State(s) to Queue__jki_lib_state_machine.vi"("State(s) in Front (\"\")"="Action: Color Table", "State(s) in (\"\")"=w298) -> ("States Out"=w297:string)  [unwired: 13 in]
          }
          event "Subtract background": Value Change {
            n157 = event-data() -> ("NewVal"=w301:bool)  [unwired: 1 in, 5 out]
            n158 = case shown="True" w301 {
              tunnel: [_ "Action: Load Background Image"] -> w302
              frame False {
              }
              frame True {
              }
            }
            n159 = call <vilib>:"Add State(s) to Queue__jki_lib_state_machine.vi"("State(s) in Front (\"\")"=w302, "State(s) in (\"\")"=w304) -> ("States Out"=w303:string)  [unwired: 13 in]
          }
          event "Scale": Value Change {
            n160 = event-data() -> ()  [unwired: 1 in, 6 out]
          }
          event "UDP error message": Value Change {
            # "popup message which is in UDP error massage"
            n161 = event-data() -> ("NewVal"=w313:string)  [unwired: 1 in, 5 out]
            n162 = Empty String/Path?(string/path=w313) -> (empty?=w314:bool)
            n163 = case shown="True" w314 {
              tunnel: w313 -> [w320 _]
              tunnel: w312 -> [w319 w321]
              tunnel: [w318 w321] -> w311
              frame False {
                n164 = call "Popup with timeout.vi"("error"=w319, "timeout"=u32 5000, "message"=w320) -> ("error out"=w318:errorcluster)  [unwired: 8 in]
              }
              frame True {
              }
            }
          }
          event "Overlay\nCentroid": Value Change {
            # "Initialize array of data size"
            n165 = event-data() -> ("NewVal"=w322:T8)  [unwired: 1 in, 5 out]
            n166 = Unbundle By Name(w322) -> ("# images to average"=w327:i32)
            n167 = Initialize Array(0.0 ("element"), w327) -> (w324:dbl[])
            n168 = Initialize Array(0.0 ("element"), w327) -> (w323:dbl[])
            n169 = Bundle By Name(cluster=w326, "Image Process.GUI_centroid overlay.CentroidX array"=w324, "Image Process.GUI_centroid overlay.CentroidY array"=w323) -> (w325:T24)
          }
          event "Draw From\n Centroid 1": Value Change {
            n170 = event-data() -> ()  [unwired: 1 in, 6 out]
            n171 = property on="centroidx::1" class="DigNum (strict)"() -> ("Value"=w336:dbl)  [unwired: 2 in, 2 out]
            n172 = property on="centroidy::1" class="DigNum (strict)"() -> ("Value"=w334:dbl)  [unwired: 2 in, 2 out]
            n173 = local write "Draw From\n Centroid 1"(FALSE ("Draw From Centroid 2")) -> ()
            n174 = To Long Integer(number=w336) -> (32bit integer=w335:i32)
            n175 = To Long Integer(number=w334) -> (32bit integer=w333:i32)
            n176 = property on="Target.X::1" class="DigNum (strict)"("Val(Sgnl)"=w335) -> ()  [unwired: 2 in, 2 out]
            n177 = property on="Target.Y::1" class="DigNum (strict)"("Val(Sgnl)"=w333) -> ()  [unwired: 2 in, 2 out]
          }
          event "Draw From Centroid 2": Value Change {
            n178 = event-data() -> ()  [unwired: 1 in, 6 out]
            n179 = property on="centroidx::1" class="DigNum (strict)"() -> ("Value"=w344:dbl)  [unwired: 2 in, 2 out]
            n180 = property on="centroidy::1" class="DigNum (strict)"() -> ("Value"=w343:dbl)  [unwired: 2 in, 2 out]
            n181 = local write "Draw From Centroid 2"(FALSE ("Draw From Centroid 2")) -> ()
            n182 = To Long Integer(number=w344) -> (32bit integer=w341:i32)
            n183 = To Long Integer(number=w343) -> (32bit integer=w342:i32)
            n184 = property on="Target2.X::1" class="DigNum (strict)"("Val(Sgnl)"=w341) -> ()  [unwired: 2 in, 2 out]
            n185 = property on="Target2.Y::1" class="DigNum (strict)"("Val(Sgnl)"=w342) -> ()  [unwired: 2 in, 2 out]
          }
        }
      }
      frame "---------- Core ----------" {
        # "Do not put any code in this frame.\n(it is a separator no-op)"
        n186 = call <vilib>:"Add State(s) to Queue__jki_lib_state_machine.vi"("State(s) in (\"\")"=w351) -> ("States Out"=w350:string)  [unwired: 14 in]
      }
      frame Default {
        w361 = 42 items=["No error", "Argument error", "Memory is full", "Out of zone", "End of file", "File already open", "Generic file I/O error", "File not found", "File permission error", "Disk is full", "Duplicate path", "Too many files open", "System feature not enabled", "Resource file not found", "Cannot add resource", "Resource not found", "Image not found", "Image memory error", "Pen does not exist", "Config type invalid", "Config token not found", "Config parse error", "Config memory error", "Bad external code format", "Bad external code offset", "External code not present", "Null window", "Destroy window error", "Null menu", "Print aborted", "Bad print record", "Print driver error", "Windows error during printing", "Memory error during printing", "Print dialog error", "Generic print error", "Invalid device refnum", "Device not found", "Device parameter error", "Device unit error", "Cannot open device", "Device call aborted", "Generic error", "Cancelled by user", "Object ID too low", "Object ID too high", "Object not in heap", "Unknown heap", "Unknown object (invalid DefProc)", "Unknown object (DefProc not in table)", "Message out of range", "Invalid (null) method", "Unknown message", "Manager call not supported", "Bad address", "Network operation in progress", "Network operation timed out", "Connection is busy", "Network attribute not supported", "Network error", "Address in use", "System out of memory", "Connection aborted", "Connection refused", "Not connected", "Already connected", "Connection closed", "Initialization error (interapplication manager)", "Bad occurrence", "Wait on unbound occurrence handler", "Occurrence queue overflow", "Datalog type conflict", "Unused", "Unrecognized type (interapplication manager)", "Memory corrupt", "Failed to make temporary DLL", "Old CIN version", "Drag socket not found", "Failed to load drop-object", "Failed to register OLE object", "Failed to release OLE object", "Format specifier type mismatch", "Unknown format specifier", "Too few format specifiers", "Too many format specifiers", "Scan failed", "Newer CIN version", "Error converting to variant", "Runtime menu error", "Password tampered", "Variant attribute not found", "Incompatible variant data type", "Event data is not available", "Event Store is not present", "Occurrence is not found", "Event Queue is not created", "Event info is not available", "Refnum passed is NULL", "Error retrieving Class GUID", "Error retrieving CoClass GUID", "Error retrieving TypeLib GUID.", "Bad built application magic bytes.", "Specific driver is different from the specific driver associated with the Logical Name.", "There is no session opened to the class driver.", "Max Error", "MAX - Error with config objects", "MAX - Error loading configuration", "MAX - Group not supported"]
        # "Current State"
        # "Do not delete, rename, or modify this frame.\n(this is used to capture unhandled states and typos)"
        # "Handle mistyped state name (developer tool)"
        n187 = Format Into String(format string="Software Exception: Unhandled State \"%s\"." ("message"), error in=w357, w352) -> (resulting string=w360:string, error out=w359:errorcluster)  [unwired: 1 in]
        n188 = call <vilib>:"Error Cluster From Error Code.vi"("show call chain? (False)"=TRUE, "error in (no error)"=w359, "error message (\"\")"=w360, "error code (0)"=w361) -> ("error out"=w358:errorcluster)  [unwired: 5 in]
        n189 = call <vilib>:"Add State(s) to Queue__jki_lib_state_machine.vi"("State(s) in (\"\")"=w356) -> ("States Out"=w355:string)  [unwired: 14 in]
      }
      frame "Initialize Core Data" {
        # "Do not delete, rename, or modify this frame.\n(this is used to determine panel behavior on exit)"
        # "originally closed?"
        # "exe?"
        # "If panel starts closed or is an EXE, then close it when we exit"
        n190 = property class="VI"() -> ("Front Panel.Open"=w370:bool)  [unwired: 2 in, 2 out]
        n191 = property class="App"() -> ("App.Kind"=w369:T12)  [unwired: 2 in, 2 out]
        n192 = control-ref of="Current VI Reference"() -> (w364:refnum<vi>)
        n193 = Not(x=w370) -> (.not. x?=w367:bool)
        n194 = Equal?(x=w369, y=T12."Run Time System" ("Application:Kind")) -> (x = y?=w363:bool)
        n195 = Or(x=w367, y=w363) -> (x .or. y?=w365:bool)
        n196 = Bundle By Name(cluster=w366, "Core.Current VI Reference"=w364, "Core.Close Panel on Exit?"=w365) -> (w372:T24)
        n197 = call <vilib>:"Add State(s) to Queue__jki_lib_state_machine.vi"("State(s) in (\"\")"=w374) -> ("States Out"=w373:string)  [unwired: 14 in]
      }
      frame "Error Handler" {
        # "Handle any errors here.\nYou can also output any states to clean-up after errors occur"
        n198 = Unbundle By Name(w376) -> ("code"=w377:i32)
        n199 = Absolute Value(x=w377) -> (abs(x)=w378:i32)
        n200 = case shown="1074396072" w378 {
          tunnel: w376 -> [w384 w386]
          tunnel: [errorcluster {"status"=FALSE, "code"=0, "source"=""} ("error out") w387] -> w375
          frame 0, Default {
            # "Unhandled Error -- Display it"
            # "Clear error"
            # "All other errors"
            n201 = call <vilib>:"General Error Handler.vi"("error in (no error)"=w384) -> ()  [unwired: 10 in, 5 out]
          }
          frame 1074396072 {
            # "Low Pass Error Code (Error occurs when image border size above 20)"
            n202 = One Button Dialog(message="Low pass size is too large. Max supported is 7x7", button name ("OK")="OK") -> (true=w385:bool)
            n203 = case shown="True" w385 {
              tunnel: [w390 errorcluster {"status"=FALSE, "code"=0, "source"=""} ("error out")] -> w387
              tunnel: w386 -> [w390 _]
              frame False {
              }
              frame True {
                # "Clear error"
                n204 = property on="LowPass" class="Bool (strict)"("Value"=FALSE ("LowPass")) -> ()  [unwired: 2 in, 2 out]
              }
            }
          }
        }
        n205 = call <vilib>:"Add State(s) to Queue__jki_lib_state_machine.vi"("State(s) in Front (\"\")"="/* Post Error States", "State(s) in (\"\")"=w382) -> ("States Out"=w381:string)  [unwired: 13 in]
      }
      frame "Exit" {
        # "Do not put any code in this frame.\n(No errors that occur here will be handled.)"
        n206 = call <vilib>:"Add State(s) to Queue__jki_lib_state_machine.vi"("State(s) in (\"\")"=w397) -> ("States Out"=w396:string)  [unwired: 14 in]
      }
      frame "---------- Data ----------" {
        # "Do not put any code in this frame.\n(It is a separator no-op. You can make a copy of this frame to create a new Data frame)"
        n207 = call <vilib>:"Add State(s) to Queue__jki_lib_state_machine.vi"("State(s) in (\"\")"=w401) -> ("States Out"=w400:string)  [unwired: 14 in]
      }
      frame "Data: Initialize" {
        w402 = 0.0  # Old Timestamp
        w403 = path ""  # PerspectivePath
        w404 = string[] []  # All Devices
        w407 = T25 7 items=["Grayscale (U8)", "Grayscale (I16)", "Grayscale (SGL)", "Complex (CSG)", "RGB (U32)", "HSL (U32)", "RGB (U64)", "Grayscale (U16)"] ("Image Type")
        w409 = dbl[][] []  # Graph
        w410 = T26 {"image::1"="image::1", "STOP queue"=refnum, "SuperGUI ref"=refnum}  # Supergui
        w411 = 0.0  # Max count before Image Processing
        w413 = 0.0  # Max count
        w414 = cluster{"size":T23, "Resize Image":bool} {"size"={"Left"=0, "Top"=0, "Right"=0, "Bottom"=0}, "Resize Image"=FALSE}  # FP
        w415 = T22 {"Analysis"={"IN"={"SpatialCalibration"=0.0, "FWHMx"=0.0, "FWHMy"=0.0, "Analysis"=FALSE}, "OUT"={"FWHMx (um)"=0.0, "FWHMy (um)"=0.0}}, "Histogram OUT"={"histogram"={"Starting Value"=0.0, "Incremental Value"=0.0, "Histogram"=[]}, "Mean Value Graph"=0.0, "Mean Value"=0.0}, "Lineout"={"IN"={"ROI"={"Global Rectangle"=[], "Contours"=[]}}, "OUT"={"lineout"={"x0"=0.0, "dx"=0.0, "Pixels Line"=[]}, "Centroid"={"X Centroid"=0.0, "Y Centroid"=0.0}, "Max Counts"={"Max"=0.0, "Color"=0}}}, "Image"=refnum, "variables"={"2ndmomW0y45::1"=0.0, "2ndmomW0x45::1"=0.0, "2ndmomW0y::1"=0.0, "2ndmomW0x::1"=0.0}}  # Image Analysis
        w416 = T21 {"Crosshair IN"={"Draw"=FALSE, "Target"={"x"=0.0, "y"=0.0}, "Size"={"x"=0.0, "y"=0.0}, "Angle"=0.0, "Color"=0, "Thickness"=0, "CrosshairLabel"=""}, "Autoscale"=FALSE, "Scale"={"scale factor"=0.0, "Scale"=FALSE}, "Lowpass IN"={"LowPass"=FALSE, "Size & Tolerance"={"X Size"=0, "Y Size"=0, "% Tolerance"=0}}, "Image"=refnum, "GUI_centroid overlay"={"CentroidX array"=[], "CentroidY array"=[], "CentroidX"=0.0, "CentroidY"=0.0, "# images to average"=0, "Crosshair"={"Draw"=FALSE, "Target"={"x"=0.0, "y"=0.0}, "Size"={"x"=0.0, "y"=0.0}, "Angle"=0.0, "Color"=0, "Thickness"=0, "CrosshairLabel"=""}}, "GUI Crosshair"={"Draw"=FALSE, "Target"={"x"=0.0, "y"=0.0}, "Size"={"x"=0.0, "y"=0.0}, "Angle"=0.0, "Color"=0, "Thickness"=0, "CrosshairLabel"=""}, "Crosshair2 IN"={"Draw"=FALSE, "Target"={"x"=0.0, "y"=0.0}, "Size"={"x"=0.0, "y"=0.0}, "Angle"=0.0, "Color"=0, "Thickness"=0, "CrosshairLabel"=""}, "calibration image"=refnum, "Perspective correection"=FALSE, "Background image"=refnum, "Subtract background"=FALSE, "Rotate Image"={"Rotate"=FALSE, "Rotation Angle"=0.0}, "Flip Image"={"Ring"=0, "Flip"=FALSE}}  # Image Process
        w419 = T25 7 items=["Grayscale (U8)", "Grayscale (I16)", "Grayscale (SGL)", "Complex (CSG)", "RGB (U32)", "HSL (U32)", "RGB (U64)", "Grayscale (U16)"] ("Image Type")
        w420 = string[] []  # subscribe messages
        w422 = T20 {"Image SM"=refnum, "valid image"=FALSE, "X resolution"=0, "Y resolution"=0, "Image Area"={"Width"=0, "Height"=0}, "zoom to fit"=FALSE, "Image Center"={"X"=0, "Y"=0}, "Max count"=0.0}  # Image Data
        w424 = T27 {"Current VI Reference"=refnum, "Close Panel on Exit?"=FALSE}  # Core
        # "Initialize the shift-register data, here.\n(data names are defined by what you wire into the bundle function)"
        n208 = call "IMAQ Create"("Border Size"=21, "Image Name"="image out", "Image Type"=w419) -> ("New Image"=w417:T1)  [unwired: 2 in, 1 out]
        n209 = call "IMAQ Create"("Border Size"=21, "Image Name"="ImageChanged", "Image Type"=w407) -> ("New Image"=w405:T1)  [unwired: 2 in, 1 out]
        n210 = Bundle By Name(cluster=w422, "Image SM"=w417) -> (w421:T20)
        n211 = Bundle("Core"=w424, "tcp connections"=refnum<k5>[] [], "subscribe messages"=w420, "Image Data"=w421, "Image Process"=w416, "Image Analysis"=w415, "FP"=w414, "Max count"=w413, "Max count before Image Processing"=w411, "Supergui"=w410, "Graph"=w409, "New Image"=w405, "All Devices"=w404, "PerspectivePath"=w403, "Old Timestamp"=w402) -> (w426:T24)  [unwired: 1 in]
        n212 = call <vilib>:"Add State(s) to Queue__jki_lib_state_machine.vi"("State(s) in (\"\")"=w428) -> ("States Out"=w427:string)  [unwired: 14 in]
      }
      frame "Data: Cleanup" {
        # "Cleanup any data and references, here.\n(this is called automatically, by the Macro: Exit)"
        n213 = Unbundle By Name(w434) -> ("Core.Current VI Reference"=w435:refnum<vi>, "Image Data.Image SM"=w433:T1)  [unwired: 2 out]
        n214 = call "IMAQ Dispose"("Image"=w433, "error in (no error)"=w430) -> ("error out"=w429:errorcluster)  [unwired: 4 in]
        n215 = disable-structure shown="Enabled" {
          disable-tunnel: w435 -> [w440 _]
          disable-tunnel: w429 -> [w439 _]
          disable-tunnel: [w438 _] -> w432
          frame Enabled {
            n216 = Close Reference(reference=w440, error in (no error)=w439) -> (error out=w438:errorcluster)
          }
          frame Disabled {
          }
        }
        n217 = call <vilib>:"Clear Errors.vi"("error in (no error)"=w432) -> ("error out"=w431:errorcluster)  [unwired: 5 in, 1 out]
        n218 = call <vilib>:"Add State(s) to Queue__jki_lib_state_machine.vi"("State(s) in (\"\")"=w437) -> ("States Out"=w436:string)  [unwired: 14 in]
      }
      frame "---------- UI ----------" {
        # "Do not put any code in this frame.\n(It is a separator no-op. You can make a copy of this frame to create a new UI frame)"
        n219 = call <vilib>:"Add State(s) to Queue__jki_lib_state_machine.vi"("State(s) in (\"\")"=w444) -> ("States Out"=w443:string)  [unwired: 14 in]
      }
      frame "UI: Initialize" {
        w452 = FALSE ("hide controls")
        w447 = u32 3 items=["Grayscale", "Binary", "Gradient", "Rainbow", "Temperature", "User Defined"] ("Palette:Palette Type")
        # "Edit mode untill Device list doesnt \nget update in runtime menu"
        # "Initialize the User Interface, here.\n(this is called automatically, by the Macro: Init)"
        n220 = property on="Scale" class="Bool (strict)"("Value"=w452) -> ()  [unwired: 2 in, 2 out]
        n221 = property on="GUI_Analysis" class="Bool (strict)"("Value"=w452) -> ()  [unwired: 2 in, 2 out]
        n222 = property on="Autoscale" class="Bool (strict)"("Value"=w452) -> ()  [unwired: 2 in, 2 out]
        n223 = property on="Scale" class="Bool (strict)"("Value"=w452) -> ()  [unwired: 2 in, 2 out]
        n224 = property on="Maximize!!" class="Bool (strict)"("Value"=w452) -> ()  [unwired: 2 in, 2 out]
        n225 = local write "Image (IMAQ)"(T1 refnum ("Image Out")) -> ()
        n226 = local write "Hide controls"(FALSE ("hide controls")) -> ()
        n227 = property on="Color table" class="Enum (strict)"("Value"=image_color_table_presets."Rainbow" ("Color table")) -> ()  [unwired: 2 in, 2 out]
        n228 = property on="Image (IMAQ)" class="ImageControl"("Palette Type"=w447) -> ()  [unwired: 2 in, 2 out]
        n229 = property on="LowPass" class="Bool (strict)"("Value"=w452) -> ()  [unwired: 2 in, 2 out]
        n230 = property on="draw Xhair" class="Bool (strict)"("Value"=TRUE ("draw Xhair")) -> ()  [unwired: 2 in, 2 out]
        n231 = control-ref of="This VI"() -> (w451:refnum<vi>)
        n232 = property on="Image (IMAQ)" class="ImageControl"("Zoom to Fit Mode"=TRUE) -> ()  [unwired: 2 in, 2 out]
        n233 = property on="Splitter" class="Splitter"("Position"=372 ("Splitter Position")) -> ()  [unwired: 2 in, 2 out]
        n234 = property class="VI"(reference=w451, "Edit Mode"=FALSE ("Edit Mode On Open")) -> ()  [unwired: 1 in, 2 out]
        n235 = Bundle By Name(cluster=w455, "Image Data.zoom to fit"=TRUE, "FP.Resize Image"=FALSE) -> (w454:T24)
        n236 = call <vilib>:"Add State(s) to Queue__jki_lib_state_machine.vi"("State(s) in (\"\")"=w461) -> ("States Out"=w460:string)  [unwired: 14 in]
      }
      frame "UI: Update Experiment Lines" {
        n237 = control-ref of="This VI"() -> (w470:refnum<vi>)
        n238 = Current VI's Menubar() -> (w472:refnum<k9>)
        n239 = call "Get list of Experiment Lines.vi"("error in (no error)"=w469, "This vi ref"=w470, "menu reference"=w472) -> ("error out"=w464:errorcluster)  [unwired: 7 in, 1 out]
        n240 = for {
          tunnel: [w475] -> w466 mode=concatenating
          tunnel: string[] ["Photometrics_CH-250_Cam", "Point Grey Camera", "Photometrics Cam", "Manta Camera", "Basler Camera", "AndorCamera", "SVimage", "MagSpecCamera", "MagSpecStitcher", "ThorLabsCsCamera", "PCO_Camera", "GEECS_Image"] -> [w474] mode=indexing
          n241 = call "getDevices.vi"("Device Class"=w474) -> ("All Devices"=w475:string[])  [unwired: 1 out]
        }
        n242 = call <vilib>:"Clear Errors.vi"("error in (no error)"=w464) -> ("error out"=w463:errorcluster)  [unwired: 5 in, 1 out]
        n243 = call "Add devices to expt line menu.vi"("error in (no error)"=w463, "All Devices"=w466, "menu reference"=w472, "This vi ref"=w470) -> ("error out"=w465:errorcluster)  [unwired: 7 in]
        n244 = Bundle By Name(cluster=w468, "All Devices"=w466) -> (w467:T24)
        n245 = Merge Errors(w465, w464) -> (w462:errorcluster)
      }
      frame "UI: Update Device List" {
        n246 = disable-structure shown="Disabled" {
          disable-tunnel: w477 -> [w483 _]
          disable-tunnel: [w482 _] -> w476
          frame Disabled {
            # "#todo this should be in database"
            n247 = Current VI's Menubar() -> (w493:refnum<k9>)
            n248 = Get Menu Item Info(7:"Devices" ("item tag"), 8:w483, 11:w493) -> (0:w486:errorcluster, 3:w491:refnum<k9>)  [unwired: 5 out]
            n249 = Set Menu Item Info(7:"Devices" ("item tag"), 8:w486, 9:TRUE ("enabled"), 11:w491) -> (0:w487:errorcluster, 3:w489:refnum<k9>)  [unwired: 3 in]
            n250 = for {
              tunnel: [w497] -> w480 mode=concatenating
              tunnel: string[] ["Photometrics_CH-250_Cam", "Point Grey Camera", "Photometrics Cam", "Manta Camera", "Basler Camera", "AndorCamera", "SVimage", "MagSpecCamera"] -> [w496] mode=indexing
              n251 = call "getDevices.vi"("Device Class"=w496) -> ("All Devices"=w497:string[])
            }
            n252 = First Call?() -> (First Call?: T/F=w495:bool)
            n253 = case shown="True" w495 {
              tunnel: w489 -> [_ w503]
              tunnel: w480 -> [_ w502]
              tunnel: w487 -> [w498 w500]
              tunnel: [w498 w499] -> w485
              frame False {
              }
              frame True {
                n254 = for {
                  tunnel: [w510] -> w504
                  tunnel: w502 -> [w508] mode=indexing
                  tunnel: w503 -> [w507]
                  tunnel: [w506] -> w501
                  tunnel: w500 -> [w505]
                  n255 = Insert Menu Items(5:"Devices" ("menu tag"), 6:w505, 7:w508, 8:w508, 9:w507) -> (0:w506:errorcluster, 3:w510:refnum<k9>)  [unwired: 1 in, 1 out]
                }
                n256 = Enable Menu Tracking(2:w501, 4:w504) -> (0:w499:errorcluster)  [unwired: 1 in, 1 out]
              }
            }
            n257 = control-ref of="This VI"() -> (w484:refnum<vi>)
            n258 = property class="VI"(reference=w484, error in=w485, "Edit Mode"=TRUE ("Edit Mode On Open")) -> (error out=w482:errorcluster)  [unwired: 1 out]
          }
          frame Enabled {
          }
        }
      }
      frame "UI: Get Device Name" {
        n259 = First Call?() -> (First Call?: T/F=w513:bool)
        n260 = case shown="True" w513 {
          tunnel: w512 -> [w516 w518]
          tunnel: [w516 w517] -> w511
          frame False {
          }
          frame True {
            n261 = disable-structure "Get Device name from control for vi mode\nand command line arg for exe" shown="RUN_TIME_ENGINE==True" {
              disable-tunnel: w518 -> [_ w520]
              disable-tunnel: [_ w519] -> w517
              frame condition #0 (active) {
                (unwired) "Bella_TopviewCCD" ("Device Name for vi mode")
                (unwired) "HPD_CCD" ("Device Name for vi mode")
                (unwired) "P1-SideView" ("Device Name for vi mode")
              }
              frame condition #1 {
                n262 = control-ref of="This Application"() -> (w525:refnum<vi>)
                n263 = property class="App"(reference=w525) -> ("App.Args"=w524:string[])  [unwired: 1 in, 2 out]
                n264 = Index Array(array=w524, index #1=1 ("index")) -> (element #1=w521:string)  [unwired: 2 in, 2 out]
                n265 = flat-sequence {
                  tunnel: [w528] -> w519
                  tunnel: w520 -> [w527]
                  tunnel: w521 -> [w526]
                  frame #0 {
                    # "Set FP title as device name"
                    n266 = control-ref of="This VI"() -> (w531:refnum<vi>)
                    n267 = Concatenate Strings(w526, "_GUI ") -> (w530:string)
                    n268 = property class="VI"(reference=w531, error in=w527, "Front Panel.Title"=w530) -> (error out=w528:errorcluster)  [unwired: 1 out]
                  }
                }
                n269 = Empty String/Path?(string/path=w521) -> (empty?=w522:bool)
                n270 = case shown="False" w522 {
                  tunnel: w521 -> [w532 _]
                  frame False {
                    n271 = local write "GUIdevice 1"(w532) -> ()
                  }
                  frame True {
                  }
                }
              }
            }
          }
        }
      }
      frame "UI: Stop SuperGUI" {
        n272 = Unbundle By Name(w538) -> ("Supergui.SuperGUI ref"=w536:refnum<vi>, "Supergui.STOP queue"=w537:refnum<queue>)
        n273 = disable-structure shown="Disabled" {
          frame Disabled {
            # "note this is for debugging"
            # "how we have stopped supergui (we should change this eventually)"
            # "kills the vi without doing exit code"
            # "what we usually do"
            # "Elsewhere we pass a queue reference into the dynamically called vis and when parent VI the shutdown code executes it closes the queue reference (destroys the queue). The clones then produce an error (e.g. from Get Queue Status) as the queue no longer exists and that error exits the dynamically called vi. Clones shutdown in this way."
            # "#todo"
            n274 = property on="stop" class="Bool (strict)"("Val(Sgnl)"=TRUE ("Value (Signaling)")) -> (error out=w541:errorcluster)  [unwired: 2 in, 1 out]
            n275 = disable-structure shown="Enabled" {
              disable-tunnel: w541 -> [w545 w546]
              disable-tunnel: [w544 w546] -> w540
              frame Enabled {
                n276 = call <userlib>:"Wait (ms)__ogtk.vi"("error in (no error)"=w545, "milliseconds to wait"=u32 5000) -> ("error out"=w544:errorcluster)  [unwired: 8 in, 1 out]
              }
              frame Disabled {
              }
            }
            n277 = disable-structure shown="Disabled" {
              disable-tunnel: _ -> [w548 _]
              disable-tunnel: w540 -> [w547 _]
              frame Disabled {
                n278 = Close Reference(reference=w548, error in (no error)=w547) -> ()  [unwired: 1 out]
              }
              frame Enabled {
              }
            }
          }
          frame Enabled {
          }
        }
        n279 = Release Queue(queue=w537, error in (no error)=w533) -> (error out=w535:errorcluster)  [unwired: 1 in, 2 out]
        n280 = call-by-ref "Wait On Asynchronous Call"(reference=w536, error in=w535) -> ("error out"=w534:errorcluster)  [unwired: 11 in, 2 out]
      }
      frame "UI: Start SuperGUI" {
        w564 = T25 0 items=["Grayscale (U8)", "Grayscale (I16)", "Grayscale (SGL)", "Complex (CSG)", "RGB (U32)", "HSL (U32)", "RGB (U64)", "Grayscale (U16)"] ("Image Type")
        # "create stop queue for supergui and its clones"
        # "can make an icon"
        # "x100 abort will be dependent on caller VI\nx80 abort will be independent of caller vi, this will abort vi when labview is closed."
        n281 = call "IMAQ Create"("Image Name"="image::1", "Image Type"=w564) -> ("New Image"=w565:T1)  [unwired: 3 in, 1 out]
        "image::1" <- w565
        n282 = disable-structure shown="Enabled" {
          disable-tunnel: w565 -> [w576 w580]
          disable-tunnel: w554 -> [w577 _]
          disable-tunnel: [w576 w579] -> w555
          disable-tunnel: [w575 _] -> w562
          disable-tunnel: [w574 _] -> w561
          disable-tunnel: [w573 _] -> w560
          disable-tunnel: [w572 _] -> w559
          disable-tunnel: [w571 _] -> w558
          frame Enabled {
            # "Network acquire image and controls"
            n283 = control-ref of="This Application"() -> (w573:refnum<vi>)
            n284 = control-ref of="This VI"() -> (w572:refnum<vi>)
            n285 = Create User Event(user event datatype=T13 {"EventEnum"=enum."new data", "Device name"="Device name"} ("New Event"), error in=w577) -> (user event=w574:refnum<user-event>, error out=w575:errorcluster)
            "tcp data event" <- w574
            n286 = Current VI's Menubar() -> (w571:refnum<k9>)
            n287 = register-events(w574) -> ()  [unwired: 2 in, 2 out]
          }
          frame Disabled {
            # "Simulation mode"
            n288 = while {
              shift-right: [w583] -> w579
              shift-left: w580 -> [w584]
              stop <- w581 stop-if-true
              # "This creates an image of a Gaussian beam"
              n289 = call "StopFGV.vi"("Command"=enum16{"set", "get", "init"}."get") -> ("Stop out"=w581:bool)  [unwired: 9 in, 1 out]
              n290 = call "2d Gaussian array.vi"() -> ("Intensity Graph"=w586:u16[][])  [unwired: 11 in]
              n291 = call "IMAQ ArrayToImage"("Image Pixels (U8)"=w586, "Image"=w584) -> ("Image Out"=w583:T1)  [unwired: 8 in, 1 out]
              n292 = Wait (ms)(milliseconds to wait=u32 1000) -> ()  [unwired: 1 out]
            }
          }
        }
        n293 = vi-ref "GUI_Master_subvi_reentrant_queues.vi"() -> (w551:refnum<vi>)
        n294 = call "supergui create stop queue.vi"() -> ("STOP Queue out"=w552:refnum<queue>)  [unwired: 11 in]
        n295 = property class="VI"(reference=w551) -> ("Path"=w550:path)  [unwired: 1 in, 2 out]
        n296 = Open VI Reference(type specifier VI Refnum (for type only)=refnum<vi> refnum, vi path=w550, options=256, error in (no error)=w554) -> (vi reference=w569:refnum<vi>, error out=w568:errorcluster)  [unwired: 2 in]
        n297 = call-by-ref "Start Asynchronous Call"(reference=w569, error in=w568, "STOP Queue in"=w552, "This Application"=w560, 8:"error in (no error)"=w562, "tcp data event"=w561, "Caller menu reference"=w558, "Caller VI ref"=w559) -> (reference out=w549:refnum<vi>, error out=w557:errorcluster)  [unwired: 5 in, 1 out]
        n298 = Bundle By Name(cluster=w553, "Supergui.image::1"=w555, "Supergui.SuperGUI ref"=w549, "Supergui.STOP queue"=w552) -> (w556:T24)
      }
      frame "UI: Cursor Set" {
        # "Argument"
        # "Set and Unset Cursor Busy.\n(Usage: \"UI: Cursor Set >> Busy|Idle\")"
        n299 = case shown="\"Idle\", Default" w587 {
          tunnel: w589 -> [w594 w596]
          tunnel: [w593 w595] -> w588
          frame "Idle", Default {
            n300 = call <vilib>:"Unset Busy.vi"("error in (no error)"=w594) -> ("error out"=w593:errorcluster)  [unwired: 10 in]
          }
          frame "Busy" {
            n301 = call <vilib>:"Set Busy.vi"("error in (no error)"=w596) -> ("error out"=w595:errorcluster)  [unwired: 9 in, 1 out]
          }
        }
        n302 = call <vilib>:"Add State(s) to Queue__jki_lib_state_machine.vi"("State(s) in (\"\")"=w592) -> ("States Out"=w591:string)  [unwired: 14 in]
      }
      frame "UI: Front Panel State" {
        # "Set Front Panel Open or Closed\n(Usage: \"UI: Front Panel State >> Open|Close\")"
        n303 = disable-structure shown="Enabled" {
          disable-tunnel: w600 -> [w607 _]
          disable-tunnel: [w606 _] -> w599
          disable-tunnel: w598 -> [w605 _]
          disable-tunnel: w597 -> [w603 _]
          frame Enabled {
            # "Argument"
            n304 = Unbundle By Name(w605) -> ("Core.Current VI Reference"=w604:refnum<vi>)
            n305 = case shown="\"Open\", Default" w603 {
              tunnel: w607 -> [w611 w624]
              tunnel: [w613 w625] -> w606
              tunnel: w604 -> [w612 w622]
              frame "Open", Default {
                n306 = property class="VI"(reference=w612, error in=w611) -> (reference out=w609:refnum<vi>, error out=w610:errorcluster, "Front Panel.Open"=w608:bool)
                n307 = case shown="True" w608 {
                  tunnel: [w616 w619] -> w613
                  tunnel: w610 -> [w615 w619]
                  tunnel: w609 -> [w614 _]
                  frame False {
                    n308 = invoke class="VI" method="FP.Open"(reference=w614, error in=w615, "Activate"=TRUE, "State"=T11."Standard") -> (error out=w616:errorcluster)  [unwired: 1 in, 4 out]
                  }
                  frame True {
                  }
                }
              }
              frame "Close" {
                n309 = property class="VI"(reference=w622, error in=w624) -> (reference out=w621:refnum<vi>, error out=w623:errorcluster, "Front Panel.Open"=w620:bool)
                n310 = disable-structure shown="Enabled" {
                  disable-tunnel: [w629 _] -> w625
                  disable-tunnel: w623 -> [w628 _]
                  disable-tunnel: w621 -> [w627 _]
                  disable-tunnel: w620 -> [w626 _]
                  frame Enabled {
                    n311 = case shown="True" w626 {
                      tunnel: [w630 w633] -> w629
                      tunnel: w628 -> [w630 w632]
                      tunnel: w627 -> [_ w631]
                      frame False {
                      }
                      frame True {
                        n312 = invoke class="VI" method="FP.Close"(reference=w631, error in=w632) -> (error out=w633:errorcluster)  [unwired: 1 in, 2 out]
                      }
                    }
                  }
                  frame Disabled {
                  }
                }
              }
            }
          }
          frame Disabled {
          }
        }
        n313 = call <vilib>:"Add State(s) to Queue__jki_lib_state_machine.vi"("State(s) in (\"\")"=w602) -> ("States Out"=w601:string)  [unwired: 14 in]
      }
      frame "---------- Macro ----------" {
        # "Do not put any code in this frame.\n(It is a separator no-op. You can make a copy of this frame to create a new Macro frame)"
        n314 = call <vilib>:"Add State(s) to Queue__jki_lib_state_machine.vi"("State(s) in (\"\")"=w637) -> ("States Out"=w636:string)  [unwired: 14 in]
      }
      frame "Macro: Initialize" {
        w638 = "Data: Initialize\nInitialize Core Data\nUI: Initialize\nUI: Update Experiment Lines\nUI: Update Device List\nUI: Get Device Name\nUI: Start SuperGUI\nUI: Front Panel State >> Open"  # Data: Initialize Initialize Core Data UI: Initialize UI: Update Experiment Lines UI: Update Device List UI: Get Device Name UI: Start SuperGUI UI: Front Panel State >> Open
        # "Initialization Macro\n(This is called once, when the VI starts)"
        n315 = call <vilib>:"Add State(s) to Queue__jki_lib_state_machine.vi"("State(s) in Front (\"\")"=w638, "State(s) in (\"\")"=w642) -> ("States Out"=w641:string)  [unwired: 13 in]
      }
      frame "Macro: valid image" {
        # "Initialization Macro\n(This is called once, when the VI starts)"
        n316 = call <vilib>:"Add State(s) to Queue__jki_lib_state_machine.vi"("State(s) in Front (\"\")"="Action: Resize FP\nAction: Set Zoom Factor\nAction: Read Controls\nAction: Read Controls 2\nAction: Display Image", "State(s) in (\"\")"=w647) -> ("States Out"=w646:string)  [unwired: 13 in]
      }
      frame "Macro: Exit" {
        # "Exit Macro\n(This is called once, when the VI exits)"
        n317 = Unbundle By Name(w657) -> ("Core.Close Panel on Exit?"=w656:bool, "Supergui.image::1"=w649:T1)
        n318 = call "IMAQ Dispose"("Image"=w649) -> ()  [unwired: 5 in, 1 out]
        n319 = Select(t="UI: Front Panel State >> Close", s=w656, f="") -> (s? t:f=w654:string)
        n320 = call <vilib>:"Add State(s) to Queue__jki_lib_state_machine.vi"("State(s) in Front (\"\")"="UI: Stop SuperGUI" ("State(s) in Front (\"\")"), "State(s) in (\"\")"=w654, "State(s) at Back (\"\")"="Data: Cleanup\nExit") -> ("States Out"=w652:string)  [unwired: 12 in]
        n321 = call <vilib>:"Add State(s) to Queue__jki_lib_state_machine.vi"("State(s) in Front (\"\")"=w652, "State(s) in (\"\")"=w659) -> ("States Out"=w658:string)  [unwired: 13 in]
      }
      frame "---------- New Category ----------" {
        # "Template Separator\n(You can make a copy of, or modify, this frame)"
        n322 = call <vilib>:"Add State(s) to Queue__jki_lib_state_machine.vi"("State(s) in (\"\")"=w663) -> ("States Out"=w662:string)  [unwired: 14 in]
      }
      frame "Action: Load Background Image" {
        # "Initialization Macro\n(This is called once, when the VI starts)"
        n323 = Empty String/Path?(string/path="BackgroundPath::1") -> (empty?=w666:bool)
        n324 = case shown="False" w666 {
          tunnel: w669 -> [w672 w691]
          tunnel: w664 -> [w689 w690]
          tunnel: [w688 w690] -> w668
          tunnel: "BackgroundPath::1" -> [w684 _]
          tunnel: [w679 w691] -> w665
          tunnel: w664 -> [w676 _]
          frame False {
            w678 = T25 7 items=["Grayscale (U8)", "Grayscale (I16)", "Grayscale (SGL)", "Complex (CSG)", "RGB (U32)", "HSL (U32)", "RGB (U64)", "Grayscale (U16)"] ("Image Type")
            n325 = Unbundle By Name(w676) -> ("Image Process.Background image"=w675:T1)
            n326 = call "IMAQ Dispose"("Image"=w675, "error in (no error)"=w672) -> ("error out"=w674:errorcluster)  [unwired: 4 in]
            n327 = call <vilib>:"Clear Errors.vi"("error in (no error)"=w674) -> ("error out"=w673:errorcluster)  [unwired: 5 in, 1 out]
            n328 = call "IMAQ Create"("Border Size"=21, "Image Name"="bg image file", "Image Type"=w678, "error in (no error)"=w673) -> ("New Image"=w686:T1, "error out"=w687:errorcluster)  [unwired: 1 out]
            n329 = call "IMAQ Read Image And Vision Info"("File Path"=w684, "error in (no error)"=w687, "Image"=w686) -> ("error out"=w680:errorcluster, "Image Out"=w682:T1)  [unwired: 1 in, 6 out]
            n330 = call "compress to 8 bit imaq cast.vi"("error in (no error)"=w680, "Image Dst Out"=w682, "Bit depth"="BG Bit depth", "Refnum in"=w682) -> ("error out"=w679:errorcluster, "Refnum out"=w681:T1)  [unwired: 6 in]
            n331 = Bundle By Name(cluster=w689, "Image Process.Background image"=w681) -> (w688:T24)
          }
          frame True {
          }
        }
        n332 = call <vilib>:"Add State(s) to Queue__jki_lib_state_machine.vi"("State(s) in (\"\")"=w671) -> ("States Out"=w670:string)  [unwired: 14 in]
      }
      frame "Action: Load Perspective Calibration" {
        n333 = Unbundle By Name(w697) -> ("PerspectivePath"=w696:path)
        n334 = Equal?(x=w696, y="PerspectivePath::1") -> (x = y?=w693:bool)
        n335 = Empty String/Path?(string/path="PerspectivePath::1") -> (empty?=w694:bool)
        n336 = Or(x=w693, y=w694) -> (x .or. y?=w692:bool)
        n337 = Bundle By Name(cluster=w697, "PerspectivePath"="PerspectivePath::1") -> (w698:T24)
        n338 = case shown="False" w692 {
          tunnel: w701 -> [w709 w711]
          tunnel: w698 -> [w707 w710]
          tunnel: [w706 w710] -> w700
          tunnel: "PerspectivePath::1" -> [w704 _]
          tunnel: [w708 w711] -> w699
          frame False {
            n339 = call "load image perspective calibration.vi"("error in (no error)"=w709, "Calibration File Path"=w704) -> ("error out"=w708:errorcluster, "Refnum out"=w705:T1)  [unwired: 8 in]
            n340 = Bundle By Name(cluster=w707, "Image Process.calibration image"=w705) -> (w706:T24)
          }
          frame True {
          }
        }
        n341 = call <vilib>:"Add State(s) to Queue__jki_lib_state_machine.vi"("State(s) in (\"\")"=w703) -> ("States Out"=w702:string)  [unwired: 14 in]
      }
      frame "Action: Load Image" {
        w718 = "image::1" ("Image Name")
        # "4/29 - Histogram now used to check\nif the image is different from old image\nas a troubleshooting indicator"
        # "4/29 - Changed Logic to the use\ntimestamps instead of just histogram difference"
        # "Max count from actual image"
        # "Is image the same?\nif yes do nothing.\nIf no then go to get image size\nIf size different then \nResize FP and set zoom factor\nIf not don't above either way\nprocess and display image"
        # "Load Image from File"
        n342 = Unbundle By Name(w725) -> ("Old Timestamp"=w716:dbl, "New Image"=w730:T1, "Image Data.Image SM"=w723:T1)
        n343 = property on="acq_timestamp::1" class="DigNum (strict)"() -> ("Value"=w715:dbl)  [unwired: 2 in, 2 out]
        n344 = call "IMAQ Histograph"("error in (no error)"=w734, "Image"=w730) -> ("error out"=w736:errorcluster, "Histogram Graph"=w731:T10)  [unwired: 6 in, 2 out]
        n345 = call <vilib>:"Clear Errors.vi"("error in (no error)"=w736) -> ("error out"=w733:errorcluster)  [unwired: 5 in, 1 out]
        n346 = call "IMAQ Histograph"("error in (no error)"=w733, "Image"=w718) -> ("error out"=w737:errorcluster, "Histogram Graph"=w738:T10)  [unwired: 6 in, 2 out]
        n347 = Greater Or Equal?(x=w715, y=w716) -> (x >= y?=w714:bool)
        n348 = Not Equal?(x=w738, y=w731) -> (x != y?=w712:bool)
        "Image Different?" <- w712
        n349 = call <vilib>:"Clear Errors.vi"("error in (no error)"=w737) -> ("error out"=w732:errorcluster)  [unwired: 5 in, 1 out]
        n350 = And(x=w714, y=w712) -> (x .and. y?=w713:bool)
        n351 = call "IMAQ Copy"("error in (no error)"=w732, "Image Dst"=w730, "Image Src"=w718) -> ("error out"=w728:errorcluster, "Image Dst Out"=w729:T1)  [unwired: 3 in]
        n352 = call "IMAQ Copy"("Image Dst"=w723, "Image Src"=w718) -> ("Image Dst Out"=w720:T1)  [unwired: 4 in, 1 out]
        n353 = case shown="True" w713 {
          tunnel: [_ "Action: Get Image Size"] -> w735
          tunnel: w729 -> [_ w759]
          tunnel: w725 -> [w746 w755]
          tunnel: w728 -> [w747 w757]
          tunnel: [w747 w756] -> w727
          tunnel: [w746 w754] -> w724
          tunnel: [w742 w748] -> w717
          tunnel: w716 -> [w742 _]
          tunnel: w715 -> [w741 w748]
          frame False {
            n354 = Get Date/Time In Seconds() -> (seconds since 1Jan1904=w744:timestamp)
            n355 = To Double Precision Float(number=w744) -> (double precision float=w743:dbl)
            n356 = Subtract(x=w743, y=w741) -> (x-y=w745:dbl)
            n357 = property on="LastUpdate(s)" class="DigNum (strict)"("Value"=w745) -> ()  [unwired: 2 in, 2 out]
          }
          frame True {
            # "image is new"
            n358 = Get Date/Time In Seconds() -> (seconds since 1Jan1904=w751:timestamp)
            n359 = call "IMAQ Histogram"("error in (no error)"=w757, "Image"=w759) -> ("error out"=w756:errorcluster, "Histogram Report"=w758:T28)  [unwired: 8 in]
            n360 = To Double Precision Float(number=w751) -> (double precision float=w750:dbl)
            n361 = Unbundle By Name(w758) -> ("Maximal Value"=w753:sgl)
            n362 = Subtract(x=w750, y=w748) -> (x-y=→"LastUpdate(s)":dbl)
            n363 = Bundle By Name(cluster=w755, "Image Data.Max count"=w753, "Max count before Image Processing"=w753) -> (w754:T24)
            n364 = To Time Stamp(1:w748) -> (0:→"Timestamp":timestamp)
          }
        }
        n365 = call "IMAQ Read Custom Data"("Key"="bitdepth", "Image"=w718) -> ("error out"=w719:errorcluster, "Custom Data Out"=→"Custom Data Out":string)  [unwired: 7 in, 1 out]
        n366 = call <vilib>:"Clear Errors.vi"("error in (no error)"=w719) -> ()  [unwired: 5 in, 2 out]
        n367 = call <vilib>:"Add State(s) to Queue__jki_lib_state_machine.vi"("State(s) in Front (\"\")"=w735, "State(s) in (\"\")"=w740) -> ("States Out"=w739:string)  [unwired: 13 in]
        n368 = Bundle By Name(cluster=w724, "Old Timestamp"=w717, "Image Data.Image SM"=w729, "New Image"=w720) -> (w726:T24)
      }
      frame "Action: Get Image Size" {
        n369 = Unbundle By Name(w771) -> ("Image Data.X resolution"=w773:i32, "Image Data.Y resolution"=w772:i32, "Image Data.Image SM"=w761:T1)
        n370 = case shown="No Error" w766 {
          selector: w766 -> [w781 w801]
          tunnel: [w782 _] -> w769
          tunnel: [w779 _] -> w768
          tunnel: w761 -> [w780 _]
          tunnel: [w775 _] -> w767
          tunnel: [w787 w801] -> w765
          tunnel: [w778 _] -> w762
          tunnel: w773 -> [w786 _]
          tunnel: w772 -> [w785 _]
          frame No Error {
            n371 = call "Get Resolution.vi"("Image"=w780, "error in (no error)"=w781) -> ("X Resolution"=w782:i32, "Y Resolution"=w779:i32, "Image Area:Size:All Elements"=w775:cluster{"Width":u32, "Height":u32}, "valid Image"=w777:bool, "error out"=w774:errorcluster)  [unwired: 9 in]
            n372 = Build Array(w786, w785) -> (w784:i32[])
            n373 = Build Array(w782, w779) -> (w783:i32[])
            n374 = Not Equal?(x=w784, y=w783) -> (x != y?=w776:bool)
            n375 = case shown="True" w777 {
              tunnel: [w788 w795] -> w787
              tunnel: w774 -> [w788 w794]
              tunnel: ["" w790] -> w778
              tunnel: w776 -> [_ w793]
              frame False {
                # "image not valid"
              }
              frame True {
                # "Image valid"
                n376 = case shown="False" w793 {
                  tunnel: [w797 w800] -> w795
                  tunnel: w794 -> [w797 w799]
                  tunnel: ["" "Action: Resize FP\nAction: Set Zoom Factor"] -> w791
                  frame False {
                    # "Image size not changed"
                  }
                  frame True {
                    # "Image res changed"
                    n377 = invoke on="Image (IMAQ)" class="ImageControl" method="FitControlToPane"(error in=w799) -> (error out=w800:errorcluster)  [unwired: 2 in, 2 out]
                  }
                }
                n378 = call <vilib>:"Add State(s) to Queue__jki_lib_state_machine.vi"("State(s) in (\"\")"=w791, "State(s) at Back (\"\")"="Action: Read Controls\nAction: Read Controls 2\nAction: Load Perspective Calibration\nAction: Process Image\nAction: Display Image") -> ("States Out"=w790:string)  [unwired: 13 in]
              }
            }
          }
          frame Error {
          }
        }
        n379 = Bundle By Name(cluster=w771, "Image Data.X resolution"=w769, "Image Data.Y resolution"=w768, "Image Data.Image Area"=w767) -> (w770:T24)
        n380 = call <vilib>:"Add State(s) to Queue__jki_lib_state_machine.vi"("State(s) in Front (\"\")"=w762, "State(s) in (\"\")"=w764) -> ("States Out"=w763:string)  [unwired: 13 in]
      }
      frame "Action: Resize FP" {
        # "Resize FP as per\nthe image size"
        # "Adjust the aspect ration as per the \nresize image height and width"
        # "Aspect ratio"
        # "Resizes Front panel as per the image size. The new vertical size is used to adjust the right panel bounds so that the panel size matches the image aspect ratio"
        n381 = disable-structure shown="Enabled" {
          disable-tunnel: w824 -> [w827 _]
          disable-tunnel: [w826 _] -> w808
          frame Enabled {
            n382 = invoke on="Image (IMAQ)" class="ImageControl" method="FitControlToPane"(error in=w827) -> (error out=w826:errorcluster)  [unwired: 2 in, 2 out]
          }
          frame Disabled {
          }
        }
        n383 = Unbundle By Name(w804) -> ("Image Data.Y resolution"=w810:i32, "Image Data.X resolution"=w809:i32)
        n384 = property on="Image (IMAQ)" class="ImageControl"(error in=w808) -> (error out=w812:errorcluster, "Image Area Height"=w822:u32, "Image Area Width"=w819:u32)  [unwired: 1 in, 1 out]
        n385 = Divide(x=w810, y=w809) -> (x/y=w823:dbl)
        n386 = control-ref of="This VI"() -> (w818:refnum<vi>)
        n387 = property class="VI"(reference=w818, error in=w812) -> (reference out=w816:refnum<vi>, error out=w811:errorcluster, "Front Panel.PanelBounds"=w817:T23)
        n388 = Divide(x=w822, y=w823) -> (x/y=w820:dbl)
        n389 = Subtract(x=w820, y=w819) -> (x-y=w821:dbl)
        n390 = Unbundle By Name(w817) -> ("Right"=w815:i16)
        n391 = To Word Integer(number=w821) -> (16bit integer=w814:i16)
        n392 = Add(x=w815, y=w814) -> (x+y=w813:i16)
        n393 = Bundle By Name(cluster=w817, "Right"=w813) -> (w802:T23)
        n394 = Bundle By Name(cluster=w804, "FP.size"=w802) -> (w803:T24)
        n395 = property class="VI"(reference=w816, error in=w811, "Front Panel.PanelBounds"=w802) -> (error out=w825:errorcluster)  [unwired: 1 out]
        n396 = call <vilib>:"Add State(s) to Queue__jki_lib_state_machine.vi"("State(s) in (\"\")"=w805) -> ("States Out"=w806:string)  [unwired: 14 in]
        n397 = call <vilib>:"Clear Errors.vi"("error in (no error)"=w825) -> ("error out"=w807:errorcluster)  [unwired: 5 in, 1 out]
      }
      frame "Action: Set Zoom Factor" {
        # "#todo the recenter image position is no longer working"
        # "Changed size of image"
        # "Calcultes zoom factor for image as per the changed size of image"
        n398 = Unbundle By Name(w835) -> ("Image Data.Image Area"=w837:cluster{"Width":u32, "Height":u32}, "Image Data.Image Center"=w830:cluster{"X":u32, "Y":u32}, "Image Data.zoom to fit"=w829:bool)
        n399 = disable-structure shown="Enabled" {
          disable-tunnel: w833 -> [w844 _]
          disable-tunnel: [w843 _] -> w832
          frame Enabled {
            n400 = invoke on="Image (IMAQ)" class="ImageControl" method="FitControlToPane"(error in=w844) -> (error out=w843:errorcluster)  [unwired: 2 in, 2 out]
          }
          frame Disabled {
          }
        }
        n401 = property on="Image (IMAQ)" class="ImageControl"(error in=w832) -> ("Image Area Size"=w841:cluster{"Width":u32, "Height":u32})  [unwired: 1 in, 2 out]
        n402 = Not Equal?(x=w837, y=w841) -> (x != y?=w842:bool)
        n403 = case shown="True" w842 {
          tunnel: w841 -> [_ w851]
          tunnel: w837 -> [_ w850]
          tunnel: [_ w846] -> w840
          frame False {
          }
          frame True {
            n404 = property on="Image (IMAQ)" class="ImageControl"() -> ("ZoomSingle"=w849:cluster{"X":sgl, "Y":sgl})  [unwired: 2 in, 2 out]
            n405 = Divide(x=w851, y=w850) -> (x/y=w847:cluster{"Width":dbl, "Height":dbl})
            n406 = Unbundle(w847) -> ("Height"=w845:dbl)  [unwired: 1 out]
            n407 = Multiply(x=w845, y=w849) -> (x*y=w848:cluster{"X":dbl, "Y":dbl})
            n408 = property on="Image (IMAQ)" class="ImageControl"("ZoomSingle"=w848) -> (error out=w846:errorcluster)  [unwired: 2 in, 1 out]
          }
        }
        n409 = property on="Image (IMAQ)" class="ImageControl"(error in=w840, "Image Center Position"=w830) -> (error out=w838:errorcluster)  [unwired: 1 in, 1 out]
        n410 = property on="Image (IMAQ)" class="ImageControl"(error in=w838, "Zoom to Fit Mode"=w829) -> (error out=w839:errorcluster)  [unwired: 1 in, 1 out]
        n411 = property on="Image (IMAQ)" class="ImageControl"(error in=w839) -> (error out=w836:errorcluster, "Image Area Size"=w828:cluster{"Width":u32, "Height":u32})  [unwired: 1 in, 1 out]
        n412 = Bundle By Name(cluster=w835, "Image Data.Image Area"=w828) -> (w834:T24)
      }
      frame "Action: Read Controls" {
        n413 = Unbundle By Name(w862) -> ("Image Data.Image SM"=w884:T1)
        n414 = Bundle("TargetSize.X::1"="TargetSize.X::1", "TargetSize.Y::1"="TargetSize.Y::1") -> (w879:T29)  [unwired: 1 in]
        n415 = Bundle By Name(cluster=T16 {"SpatialCalibration"=0.0, "FWHMx"=0.0, "FWHMy"=0.0, "Analysis"=FALSE} ("Image Process.Analysis.IN"), "Analysis"="GUI_Analysis", "SpatialCalibration"="SpatialCalibration::1", "FWHMx"="FWHMx::1", "FWHMy"="FWHMy::1") -> (w883:T16)
        n416 = Bundle By Name(cluster=T17 {"LowPass"=FALSE, "Size & Tolerance"={"X Size"=0, "Y Size"=0, "% Tolerance"=0}} ("Image Process.Lowpass IN"), "LowPass"="LowPass", "Size & Tolerance"="Size & Tolerance") -> (w890:T17)
        n417 = Bundle By Name(cluster=cluster{"scale factor":dbl, "Scale":bool} {"scale factor"=0.0, "Scale"=FALSE} ("Image Process.Scale"), "scale factor"="scale factor", "Scale"="Scale") -> (w894:cluster{"scale factor":dbl, "Scale":bool})
        n418 = Bundle By Name(cluster=T9 {"Draw"=TRUE, "Target"={"x"=0.0, "y"=0.0}, "Size"={"x"=20.0, "y"=20.0}, "Angle"=0.0, "Color"=1250067, "Thickness"=0, "CrosshairLabel"=""} ("Image Process.Crosshair IN"), "Draw"="draw Xhair", "Size"=w879, "Target.x"="Target.X::1", "Target.y"="Target.Y::1", "Color"="Crosshair\nColor", "Thickness"="Crosshair Thickness", "CrosshairLabel"="Crosshair.Label1::1") -> (w857:T9)
        n419 = property on="Image (IMAQ)" class="ImageControl"() -> ("ROI"=w882:T18)  [unwired: 2 in, 2 out]
        n420 = property on="2ndmomW0x::1" class="DigNum (strict)"() -> ("Value"=w876:dbl)  [unwired: 2 in, 2 out]
        n421 = property on="2ndmomW0y::1" class="DigNum (strict)"() -> ("Value"=w875:dbl)  [unwired: 2 in, 2 out]
        n422 = property on="2ndmomW0x45::1" class="DigNum (strict)"() -> ("Value"=w874:dbl)  [unwired: 2 in, 2 out]
        n423 = property on="2ndmomW0y45::1" class="DigNum (strict)"() -> ("Value"=w873:dbl)  [unwired: 2 in, 2 out]
        n424 = Unbundle By Name("Overlay\nCentroid") -> ("draw Xhair 2"=w867:bool, "Size x"=w870:dbl, "Size y"=w869:dbl, "# images to average"=w865:i32, "Centroid \nOverlay Color"=w864:u32)
        n425 = Bundle By Name(cluster=T15 {"2ndmomW0y45::1"=0.0, "2ndmomW0x45::1"=0.0, "2ndmomW0y::1"=0.0, "2ndmomW0x::1"=0.0} ("Image Analysis.variables"), "2ndmomW0x::1"=w876, "2ndmomW0y45::1"=w875, "2ndmomW0x45::1"=w874, "2ndmomW0y::1"=w873) -> (w877:T15)
        n426 = Bundle("Size x"=w870, "Size y"=w869) -> (w866:cluster{"Size x":dbl, "Size y":dbl})  [unwired: 1 in]
        n427 = Bundle By Name(cluster=T14 {"CentroidX array"=[], "CentroidY array"=[], "CentroidX"=0.0, "CentroidY"=0.0, "# images to average"=1250067, "Crosshair"={"Draw"=FALSE, "Target"={"x"=0.0, "y"=0.0}, "Size"={"x"=0.0, "y"=0.0}, "Angle"=0.0, "Color"=0, "Thickness"=0, "CrosshairLabel"=""}} ("Image Process.GUI_centroid overlay"), "Crosshair.Draw"=w867, "Crosshair.Size"=w866, "# images to average"=w865, "Crosshair.Color"=w864, "CentroidX"="centroidx::1", "CentroidY"="centroidy::1") -> (w863:T14)
        n428 = Bundle By Name(cluster=w862, "Image Process.Image"=w884, "Image Process.Crosshair IN"=w857, "Image Process.Autoscale"="Autoscale", "Image Process.Scale"=w894, "Image Process.Lowpass IN"=w890, "Image Analysis.Analysis.IN"=w883, "Image Analysis.Lineout.IN.ROI"=w882, "Image Analysis.variables"=w877, "Image Process.GUI_centroid overlay"=w863, "Image Process.GUI Crosshair"="GUI Crosshair") -> (w899:T24)
      }
      frame "Action: Read Controls 2" {
        # "Crosshair 2"
        n429 = Bundle("Target2.X::1"="Target2.X::1", "Target2.Y::1"="Target2.Y::1") -> (w919:cluster{"Target2.X::1":dbl, "Target2.Y::1":dbl})  [unwired: 1 in]
        n430 = Bundle("Target2Size.X::1"="Target2Size.X::1", "Target2Size.Y::1"="Target2Size.Y::1") -> (w916:T30)  [unwired: 1 in]
        n431 = Bundle("Rotate"="Rotate", "Angle"="Angle") -> (w910:cluster{"Rotate":bool, "Angle":dbl})  [unwired: 1 in]
        n432 = Bundle("Type of Symmetry"="Type of Symmetry", "Rotate 2"="Rotate 2") -> (w904:T31)  [unwired: 1 in]
        n433 = Bundle By Name(cluster=w921, "Image Process.Crosshair2 IN.Draw"="draw Xhair 2", "Image Process.Crosshair2 IN.Target"=w919, "Image Process.Crosshair2 IN.Size"=w916, "Image Process.Crosshair2 IN.Color"="Crosshair 2\nColor", "Image Process.Crosshair2 IN.Thickness"="Crosshair 2Thickness", "Image Process.Crosshair2 IN.CrosshairLabel"="Crosshair.Label2::1", "Image Process.Perspective correection"="PerspectiveCorrectGUI::1", "Image Process.Subtract background"="Subtract background", "Image Process.Rotate Image"=w910, "Image Process.Flip Image"=w904) -> (w920:T24)
      }
      frame "Action: Process Image" {
        # "GUI running average centroid overlay added by Aalhad (18/6/2017)"
        n434 = local read "meancounts::1"() -> (w935:dbl)
        n435 = Unbundle By Name(w944) -> ("Image Analysis.Analysis.OUT.FWHMx (um)"=w932:dbl, "Image Analysis.Analysis.OUT.FWHMy (um)"=w933:dbl, "Image Analysis.variables.2ndmomW0x::1"=w940:dbl, "Image Analysis.variables.2ndmomW0y::1"=w939:dbl, "Image Analysis.variables.2ndmomW0x45::1"=w938:dbl, "Image Analysis.variables.2ndmomW0y45::1"=w937:dbl)
        n436 = Unbundle By Name(w944) -> ("Graph"=w942:dbl[][])
        n437 = Unbundle By Name(w944) -> ("Image Process"=w951:T21, "Image Analysis"=w946:T22)
        n438 = To Double Precision Float(number=w935) -> (double precision float=w936:dbl)
        n439 = Build Array(w932, w933, w940, w939, w938, w937, "maxcounts::1", w936, "MeanCountsRaw::1") -> (w943:dbl[])
        n440 = local read "Sat Level"() -> (w926:sgl)
        n441 = Build Array (concatenate)(w942, w943) -> (→"Chart":dbl[][])
        n442 = call <userlib>:"Tick Count (ms)__ogtk.vi"("error in (no error)"=w948) -> ("error out"=w931:errorcluster, "millisecond timer value"=w928:u32)  [unwired: 9 in]
        n443 = call "Process Image.vi"("error in (no error)"=w931, "Saturation (counts)"=w926, "Image Analysis IN"=w946, "Cluster in"=w951) -> ("error out"=w947:errorcluster, "Perspective correction error"=→"Perspective error":bool, "Image Analysis OUT"=w945:T22, "Cluster out"=w950:T21)  [unwired: 4 in]
        n444 = call <userlib>:"Tick Count (ms)__ogtk.vi"("error in (no error)"=w947) -> ("error out"=w930:errorcluster, "millisecond timer value"=w929:u32)  [unwired: 9 in]
        n445 = Subtract(x=w929, y=w928) -> (x-y=→"process time":u32)
        n446 = Bundle By Name(cluster=w944, "Image Process"=w950, "Image Analysis"=w945) -> (w949:T24)
      }
      frame "Action: Display Image" {
        # "Max count before and after image processing is added by Aalhad"
        n447 = Unbundle By Name(w972) -> ("Image Analysis.Analysis.IN.SpatialCalibration"=w960:dbl, "Image Process.Image"=w953:T1, "Image Analysis.Lineout.OUT"=w988:T32, "Image Analysis.Histogram OUT"=w987:T33, "Image Analysis.Analysis.OUT"=w984:cluster{"FWHMx (um)":dbl, "FWHMy (um)":dbl}, "Image Process.Crosshair IN.Draw"=w981:bool, "Image Process.Crosshair IN.Target.x"=w979:dbl, "Image Process.Crosshair IN.Target.y"=w978:dbl, "Max count before Image Processing"=w973:dbl)  [unwired: 1 out]
        "Image (IMAQ)" <- w953
        n448 = call "IMAQ Histogram"("error in (no error)"=w965, "Image"=w953) -> ("error out"=w966:errorcluster, "Histogram Report"=w968:T28)  [unwired: 8 in]
        n449 = Unbundle By Name(w968) -> ("Maximal Value"=w967:sgl)
        n450 = case shown="\"Before Image Processing\"" "Max count" {
          tunnel: [w990 w991] -> w974
          tunnel: w967 -> [w990 _]
          tunnel: w973 -> [_ w991]
          frame "After Image Processing", Default {
          }
          frame "Before Image Processing" {
          }
        }
        "Max Counts" <- w974
        n451 = call-poly <userlib>:"Data Changed__ogtk.vi"("Boolean"=w981) -> ("Changed"=w980:bool)
        n452 = Divide(x=w960, y=1000.0) -> (x/y=w956:dbl)
        n453 = Unbundle By Name(w988) -> ("lineout"=w964:cluster{"x0":sgl, "dx":sgl, "Pixels Line":sgl[]})  [unwired: 1 out]
        "lineout" <- w964
        n454 = Unbundle By Name(w987) -> ("histogram"=→"histogram":T10, "Mean Value"=→"Mean Value":sgl)  [unwired: 1 out]
        n455 = case shown="True" w980 {
          tunnel: w979 -> [_ w994]
          tunnel: w978 -> [_ w993]
          frame False {
          }
          frame True {
            n456 = Bundle("x"=w994, "y"=w993) -> (w992:cluster{"x":dbl, "y":dbl})  [unwired: 1 in]
            n457 = property on="Image (IMAQ)" class="ImageControl"("Image Center Position"=w992) -> ()  [unwired: 2 in, 2 out]
          }
        }
        n458 = Unbundle By Name(w984) -> ("FWHMx (um)"=→"FWHMx (um)":dbl, "FWHMy (um)"=→"FWHMy (um)":dbl)
        n459 = call "ColorRamp_TS.vi"("max value"=256, "value"=w974) -> ("Color"=w976:u32)  [unwired: 9 in]
        n460 = property on="Max Counts" class="Slide (strict)"("Fill Color"=w976) -> ()  [unwired: 2 in, 2 out]
        n461 = Unbundle(w964) -> ("Pixels Line"=w963:sgl[])  [unwired: 2 out]
        n462 = Array Size(array=w963) -> (size(s)=w962:i32)
        n463 = Divide(x=w962, y=2) -> (x/y=w957:dbl)
        n464 = Multiply(x=w956, y=w957) -> (x*y=w955:dbl)
        n465 = Tick Count (ms)() -> (millisecond timer value=w970:u32)
        n466 = Negate(x=w955) -> (-x=w958:dbl)
        n467 = feedback-in #2(w970) -> ()
        n468 = feedback #2(w970) -> (w971:u32)
        n469 = Subtract(x=w970, y=w971) -> (x-y=→"ms since last display":u32)
        n470 = property on="lineout" class="WFGraph (strict)"("XScale.Multiplier"=w956, "XScale.Offset"=w958) -> (error out=w954:errorcluster)  [unwired: 2 in, 1 out]
        n471 = call <vilib>:"Clear Errors.vi"("error in (no error)"=w954) -> ()  [unwired: 5 in, 2 out]
      }
      frame "Action: Color Table" {
        # "Chech whether user input for color table\nother than Ni pallete"
        # "When user cancels the make new one color table \nthen color table value changed to rainbow"
        n472 = property on="Color table" class="Enum (strict)"() -> ("Strings []"=w999:string[])  [unwired: 2 in, 2 out]
        n473 = Format Into String("Color table") -> (resulting string=w1000:string)  [unwired: 3 in, 1 out]
        n474 = call "IMAQ color table presets.vi"("Color table"="Color table") -> ("Make new one cancelled"=w995:bool, "Array"=w1004:cluster{"R":u8, "G":u8, "B":u8}[])  [unwired: 9 in]
        n475 = Search 1D Array(1D array=w999, element=w1000) -> (index of element=w997:i32)  [unwired: 1 in]
        n476 = Greater Or Equal?(x=w997, y=5) -> (x >= y?=w998:bool)
        n477 = case shown="True" w998 {
          tunnel: w1004 -> [_ w1013]
          tunnel: "Color table" -> [w1009 _]
          tunnel: w1003 -> [w1008 w1010]
          tunnel: [w1007 w1012] -> w1002
          tunnel: w995 -> [_ w1011]
          frame False {
            n478 = property on="Image (IMAQ)" class="ImageControl"(error in=w1008, "Palette Type"=w1009) -> (error out=w1007:errorcluster)  [unwired: 1 in, 1 out]
          }
          frame True {
            w1014 = u32 5 items=["Grayscale", "Binary", "Gradient", "Rainbow", "Temperature", "User Defined"] ("Palette:Palette Type")
            n479 = case shown="True" w1011 {
              tunnel: w1010 -> [_ w1015]
              frame False {
              }
              frame True {
                n480 = property on="Color table" class="Enum (strict)"(error in=w1015, "Val(Sgnl)"=image_color_table_presets."Rainbow" ("Value (Signaling)")) -> ()  [unwired: 1 in, 2 out]
              }
            }
            n481 = property on="Image (IMAQ)" class="ImageControl"(error in=w1010, "Palette Type"=w1014, "User Palette"=w1013) -> (error out=w1012:errorcluster)  [unwired: 1 in, 1 out]
          }
        }
      }
      frame "Action: Beep If Saturation" {
        n482 = Unbundle By Name(w1020) -> ("Image Analysis.Lineout.OUT.Max Counts.Max"=w1019:sgl)
        n483 = call "Beep if saturation.vi"("error in"=w1018, "Sat Level"="Sat Level", "Beep If Sat."="Scale", "Max"=w1019) -> ("error out"=w1017:errorcluster)  [unwired: 7 in]
      }
      frame "Action: Hide Controls" {
        w1040 = u32 0 items=["Visible", "Hidden", "Hidden, Use WindTools Palette"] ("ROI Tools Visible")
        # "As the user hide and show controls we need to resize the \npanel by adding and subtracting certain number to \"Right\" FP Bounds. The minimum pane size should be set as per the below: \n\n1. Left - Right = Width (877)\n2. Top - Bottom = Height (500)"
        # "As per the tab size splitter position is set"
        # "Hide splitter"
        n484 = Unbundle By Name(w1037) -> ("Image Data.Image Area"=w1050:cluster{"Width":u32, "Height":u32})
        n485 = Not(x="Hide controls") -> (.not. x?=w1025:bool)
        n486 = local write "Hide controls"(w1025) -> ()
        n487 = case shown="True" w1025 {
          tunnel: [372 ("Position:Left") w1060] -> w1049
          tunnel: w1027 -> [w1058 w1062]
          tunnel: [w1057 w1061] -> w1026
          frame False {
            w1059 = u32 12369084 ("Color")
            n488 = property on="Splitter" class="Splitter"(error in=w1058, "FGColor"=w1059, "BGColor"=w1059) -> (error out=w1057:errorcluster)  [unwired: 1 in, 1 out]
          }
          frame True {
            w1060 = 2 ("Position:Left")
            w1063 = u32 14869218 ("Color")
            n489 = property on="Splitter" class="Splitter"("Position"=w1060) -> ()  [unwired: 2 in, 2 out]
            n490 = property on="Splitter" class="Splitter"(error in=w1062, "FGColor"=w1063, "BGColor"=w1063) -> (error out=w1061:errorcluster)  [unwired: 1 in, 1 out]
          }
        }
        n491 = property on="Image (IMAQ)" class="ImageControl"() -> ("ROI Tools Visible"=w1041:u32)  [unwired: 2 in, 2 out]
        n492 = property class="VI"(error in=w1026) -> (error out=w1032:errorcluster, "Front Panel.WinBounds"=w1034:T23)  [unwired: 1 in, 1 out]
        n493 = Equal?(x=w1041, y=w1040) -> (x = y?=w1039:bool)
        n494 = Unbundle By Name(w1034) -> ("Right"=w1031:i16)
        n495 = property on="Image (IMAQ)" class="ImageControl"(error in=w1032, "Image Area Size"=w1050, "Zoom to Fit Mode"=FALSE) -> (error out=w1046:errorcluster)  [unwired: 1 in, 1 out]
        n496 = Select(t=420 ("Position:Left"), s=w1039, f=390 ("Position:Left")) -> (s? t:f=w1030:i32)
        n497 = Subtract(x=w1031, y=w1030) -> (x-y=w1044:i32)
        n498 = Add(x=w1030, y=w1031) -> (x+y=w1043:i32)
        n499 = Select(t=w1044, s=w1025, f=w1043) -> (s? t:f=w1042:i32)
        n500 = invoke on="Image (IMAQ)" class="ImageControl" method="FitControlToPane"(error in=w1046) -> (error out=w1033:errorcluster)  [unwired: 2 in, 2 out]
        n501 = Bundle By Name(cluster=w1034, "Right"=w1042) -> (w1045:T23)
        n502 = property class="VI"(error in=w1033, "Front Panel.WinBounds"=w1045) -> (error out=w1024:errorcluster)  [unwired: 1 in, 1 out]
        n503 = case shown="False" w1025 {
          tunnel: w1049 -> [w1054 _]
          tunnel: [w1053 w1055] -> w1028
          tunnel: w1024 -> [w1052 w1055]
          frame False {
            n504 = property on="Splitter" class="Splitter"(error in=w1052, "Position"=w1054) -> (error out=w1053:errorcluster)  [unwired: 1 in, 1 out]
          }
          frame True {
          }
        }
        n505 = invoke on="Image (IMAQ)" class="ImageControl" method="FitControlToPane"(error in=w1028) -> (error out=w1029:errorcluster)  [unwired: 2 in, 2 out]
        n506 = call <vilib>:"Add State(s) to Queue__jki_lib_state_machine.vi"("State(s) in (\"\")"=w1048) -> ("States Out"=w1047:string)  [unwired: 14 in]
      }
    }
  }
